vi "rio 9030 2.vi"() -> ()   [LabVIEW 2015]
uses:
  <vilib>/FPGAPlugInAG/cRIO-9030/niLvFpga_Open_cRIO-9030.vi
  <vilib>/rvi/interface/common/dynamic/niFpgaDynamicAddResources.vi
  <vilib>/FPGAPlugInAG/Dynamic/niLvFpga_Abort_Dynamic.vi
  <vilib>/FPGAPlugInAG/Dynamic/niLvFpga_Run_Dynamic.vi
  rio_Global.vi
  <vilib>/Utility/error.llb/Error Cluster From Error Code.vi
  <vilib>/rvi/errors/niLvFpgaAdjustHostInterfaceError.vi
  <vilib>/Analysis/Matrix/Numeric/Conversions/Array To Matrix - RA2.vi
  <vilib>/Analysis/Matrix/Numeric/Multiply/Multiply - RM,RM.vi
  <vilib>/Analysis/Matrix/Numeric/Add/Add - RM,RM.vi
  <vilib>/Analysis/baseanly.llb/Real Inverse Matrix.vi
  <vilib>/Analysis/Matrix/Numeric/Subtract/Subtract - RM,RM.vi
  <vilib>/Analysis/Matrix/Numeric/Conversions/Array To Matrix - RA.vi
  <vilib>/Analysis/Matrix/Numeric/Multiply/Multiply - R,RM.vi
  <vilib>/Analysis/Matrix/Numeric/Conversions/Matrix To Array - RM.vi
  <vilib>/rvi/interface/nirviOpenFPGA/nirviOpenFPGA.xnode
  FPGA Bitfiles/autonomous_FPGATarget4_fpga1_rudp+OsNkSQ.lvbitx
  samsung/fpga 1.vi
  <vilib>/rvi/interface/nirviMethod/nirviMethod.xnode
  <vilib>/rvi/interface/nirviReadWriteControl/nirviReadWriteControl.xnode
  <vilib>/FPGAPlugInAG/Dynamic/niLvFpga_ReadFifo_Dynamic.vi
  <vilib>/rvi/errors/niLvFpgaMergeErrorWithErrorCode.vi
  <vilib>/Analysis/Matrix/NI_Matrix.lvlib
  <vilib>/Analysis/NI_AALBase.lvlib
  <vilib>/rvi/interface/Simulation/niFpgaSimulationCallBeginRW.vi
  NiFpgaLv.dll
  <vilib>/addons/control/pid/NI_PID_pid.lvlib
  <vilib>/ptbypt/NI_PtbyPt.lvlib
  <vilib>/addons/control/pid/pid.llb/PID (DBL).vi
panel:
  in  "steering torque":dbl min=-1.0 max=1.0 step=0.1
  in  "map name":T1(ring)=enum."KAIST"
  out "Waveform Chart 3":dbl(graph)
  in  "lpf gain 2":dbl=0.8 format="%#_13g"
  out "con_dt":dbl
  in  "lpf gain":dbl=0.8 format="%#_13g"
  in  "d gain":dbl=0.003
  out "Waveform Chart 2":dbl(graph)
  in  "Dial":dbl(knob) min=-360.0 max=360.0 step=5.0 scale=-360.0..360.0
  in  "i gain":dbl=6.5
  in  "p gain":dbl=0.02
  out "FPGA":refnum<k20>
  out "C_yaw_rate":dbl
  in  "speed control":bool
  out "C_MCP":dbl
  out "C_APV":dbl
  in  "PWM GAS 2":dbl=1000.0 min=1000.0 max=2000.0 step=1.0
  out "Ref_VS":dbl
  out "XY Graph":cluster{"Y":dbl[], "Y":dbl[]}[](graph)=[{"Y"=[1.82421875, 1.8301353427767753, 1.835194070339203, 1.8394013252854347, 1.8427635002136231, 1.84528698772192, 1.8469781804084777, 1.8478434708714486, 1.8478892517089844, 1.8471219155192375, 1.84554785490036, 1.8431734624505043, 1.8400051307678222, 1.8360492524504661, 1.8313122200965881, 1.8258004263043404, 1.819520263671875, 1.8124781247973443, 1.8046804022789003, 1.796133488714695, 1.7868437767028809, 1.77681765884161, 1.7660615277290344, 1.7545817759633064, 1.742384796142578, 1.7294769808650017, 1.7158647227287291, 1.701554414331913, 1.686552448272705, 1.6708652171492577, 1.654499113559723, 1.637460530102253, 1.619755859375, 1.6013914939761162, 1.5823738265037537, 1.5627092495560646, 1.5424041557312012, 1.5214649376273155, 1.4998979878425598, 1.4777096989750862, 1.4549064636230469, 1.431494674384594, 1.4074807238578795, 1.3828710046410562, 1.3576719093322753, 1.3318898305296898, 1.3055311608314515, 1.2786022928357124, 1.251109619140625, 1.2230595323443412], "Y"=[0.0, 0.5, 1.0, 1.5, 2.0, 2.5, 3.0, 3.5, 4.0, 4.5, 5.0, 5.5, 6.0, 6.5, 7.0, 7.5, 8.0, 8.5, 9.0, 9.5, 10.0, 10.5, 11.0, 11.5, 12.0, 12.5, 13.0, 13.5, 14.0, 14.5, 15.0, 15.5, 16.0, 16.5, 17.0, 17.5, 18.0, 18.5, 19.0, 19.5, 20.0, 20.5, 21.0, 21.5, 22.0, 22.5, 23.0, 23.5, 24.0, 24.5]}, {"Y"=[-1.22265625, -1.2167396572232247, -1.211680929660797, -1.2074736747145653, -1.2041114997863769, -1.20158801227808, -1.1998968195915223, -1.1990315291285514, -1.1989857482910156, -1.1997530844807625, -1.20132714509964, -1.2037015375494957, -1.2068698692321778, -1.2108257475495339, -1.2155627799034119, -1.2210745736956596, -1.227354736328125, -1.2343968752026557, -1.2421945977210997, -1.250741511285305, -1.2600312232971191, -1.27005734115839, -1.2808134722709656, -1.2922932240366936, -1.304490203857422, -1.3173980191349983, -1.3310102772712709, -1.345320585668087, -1.360322551727295, -1.3760097828507423, -1.392375886440277, -1.409414469897747, -1.427119140625, -1.4454835060238838, -1.4645011734962463, -1.4841657504439354, -1.5044708442687988, -1.5254100623726845, -1.5469770121574402, -1.5691653010249138, -1.5919685363769531, -1.615380325615406, -1.6393942761421205, -1.6640039953589438, -1.6892030906677247, -1.7149851694703102, -1.7413438391685485, -1.7682727071642876, -1.795765380859375, -1.8238154676556588, -1.8524165749549866, -1.8815623101592065, -1.911246280670166, -1.9414620938897134, -1.972203357219696, -2.003463678061962, -2.0352366638183597, -2.0675159218907355, -2.1002950596809384, -2.1335676845908162, -2.167327404022217, -2.2015678253769875, -2.2362825560569766, -2.2714652034640315, -2.307109375, -2.3432086780667305, -2.3797567200660703, -2.4167471083998677, -2.4541734504699706, -2.4920293536782263, -2.530308425426483, -2.5690042731165885, -2.6081105041503907, -2.647620725929737, -2.687528545856476, -2.7278275713324547, -2.7685114097595216, -2.809573668539524, -2.8510079550743104, -2.892807876765728, -2.934967041015625, -2.977479055225849, -3.020337526798248, -3.0635360631346704, -3.107068271636963, -3.150927759706974, -3.1951081347465515, -3.2396030041575434, -3.284405975341797, -3.3295106557011604, -3.3749106526374817, -3.4205995735526087, -3.466571025848389, -3.51281861692667, -3.5593359541893004], "Y"=[0.0, 0.5, 1.0, 1.5, 2.0, 2.5, 3.0, 3.5, 4.0, 4.5, 5.0, 5.5, 6.0, 6.5, 7.0, 7.5, 8.0, 8.5, 9.0, 9.5, 10.0, 10.5, 11.0, 11.5, 12.0, 12.5, 13.0, 13.5, 14.0, 14.5, 15.0, 15.5, 16.0, 16.5, 17.0, 17.5, 18.0, 18.5, 19.0, 19.5, 20.0, 20.5, 21.0, 21.5, 22.0, 22.5, 23.0, 23.5, 24.0, 24.5, 25.0, 25.5, 26.0, 26.5, 27.0, 27.5, 28.0, 28.5, 29.0, 29.5, 30.0, 30.5, 31.0, 31.5, 32.0, 32.5, 33.0, 33.5, 34.0, 34.5, 35.0, 35.5, 36.0, 36.5, 37.0, 37.5, 38.0, 38.5, 39.0, 39.5, 40.0, 40.5, 41.0, 41.5, 42.0, 42.5, 43.0, 43.5, 44.0, 44.5, 45.0, 45.5, 46.0, 46.5, 47.0]}, {"Y"=[-0.94, 0.94, 0.94, -0.94, -0.94], "Y"=[-3.2, -3.2, 1.5, 1.5, -3.2]}, {"Y"=[1.984375, 1.978057861328125, 1.9718017578125, 1.965606689453125, 1.95947265625], "Y"=[0.0, 0.5, 1.0, 1.5, 2.0]}, {"Y"=[-5.28125, -5.267578125, -5.25390625, -5.240234375, -5.2265625], "Y"=[0.0, 0.5, 1.0, 1.5, 2.0]}]
  out "x_view":dbl[](array[numeric])=[0.0, 0.5, 1.0, 1.5, 2.0, 2.5, 3.0, 3.5, 4.0, 4.5, 5.0, 5.5, 6.0, 6.5, 7.0, 7.5, 8.0, 8.5, 9.0, 9.5, 10.0, 10.5, 11.0, 11.5, 12.0, 12.5, 13.0, 13.5, 14.0, 14.5, 15.0, 15.5, 16.0, 16.5, 17.0, 17.5, 18.0, 18.5, 19.0, 19.5, 20.0, 20.5, 21.0, 21.5, 22.0, 22.5, 23.0, 23.5, 24.0, 24.5, 25.0, 25.5, 26.0, 26.5, 27.0, 27.5, 28.0, 28.5, 29.0, 29.5, 30.0, 30.5, 31.0, 31.5, 32.0, 32.5, 33.0, 33.5, 34.0, 34.5, 35.0, 35.5, 36.0, 36.5, 37.0, 37.5, 38.0, 38.5, 39.0, 39.5, 40.0, 40.5, 41.0, 41.5, 42.0, 42.5, 43.0, 43.5, 44.0, 44.5, 45.0, 45.5, 46.0, 46.5, 47.0, 47.5, 48.0, 48.5, 49.0, 49.5, 50.0, 50.5, 51.0, 51.5, 52.0, 52.5, 53.0, 53.5, 54.0, 54.5, 55.0, 55.5, 56.0, 56.5, 57.0, 57.5, 58.0, 58.5, 59.0, 59.5, 60.0, 60.5, 61.0, 61.5, 62.0, 62.5, 63.0, 63.5, 64.0, 64.5, 65.0, 65.5, 66.0, 66.5, 67.0, 67.5, 68.0, 68.5, 69.0, 69.5, 70.0, 70.5, 71.0, 71.5, 72.0, 72.5, 73.0, 73.5, 74.0, 74.5, 75.0, 75.5, 76.0, 76.5, 77.0, 77.5, 78.0, 78.5, 79.0, 79.5, 80.0, 80.5, 81.0, 81.5, 82.0, 82.5, 83.0, 83.5, 84.0, 84.5, 85.0, 85.5, 86.0, 86.5, 87.0, 87.5, 88.0, 88.5, 89.0, 89.5, 90.0, 90.5, 91.0, 91.5, 92.0, 92.5, 93.0, 93.5, 94.0, 94.5, 95.0, 95.5, 96.0, 96.5, 97.0, 97.5, 98.0, 98.5, 99.0, 99.5, 100.0, 100.5, 101.0, 101.5, 102.0, 102.5, 103.0, 103.5, 104.0, 104.5, 105.0, 105.5, 106.0, 106.5, 107.0, 107.5, 108.0, 108.5, 109.0, 109.5, 110.0, 110.5, 111.0, 111.5, 112.0, 112.5, 113.0, 113.5, 114.0, 114.5, 115.0, 115.5, 116.0, 116.5, 117.0, 117.5, 118.0, 118.5, 119.0, 119.5, 120.0, 120.5, 121.0, 121.5, 122.0, 122.5, 123.0, 123.5, 124.0, 124.5, 125.0, 125.5, 126.0, 126.5, 127.0, 127.5, 128.0]
  in  "Manual Steering torque":dbl(slide) min=-0.9 max=0.9 step=0.01 scale=-0.9..0.9
  out "T init":i32
  out "T out":i32
  out "PWM GAS":dbl=1000.0 min=1000.0 max=2000.0 step=1.0
  out "Mobileye_time 50":u32
  out "H_GPS":dbl
  out "vgain":dbl=1.0
  out "vcount":u64=1
  out "hbias":dbl
  out "hcount":u64=1
  out "get heading":bool
  out "get position":bool
  out "heading error":dbl
  out "h_gps":dbl
  out "rt":dbl
  out "pos error":dbl
  out "POS init":bool
  out "Heading":dbl
  out "pos":dbl[](array[numeric])
  in  "GPS init":bool=TRUE
  out "pos_gps":dbl[](array[numeric]) format="%#_19f"
  out "dt":dbl
  out "Pos_time 10":i32
  out "map":i32=2
  out "ecef ref":dbl[](array[numeric])
  in  "Velocity input":bool
  in  "Manual Speed":dbl=20.0
  in  "Steer input":bool=TRUE
  out "Run":bool
  out "Auto":bool
  out "E - STOP":bool
  out "Con_time 10":i32
  out "VS_CAN":dbl
  out "CAN_time 10":u32
  out "gps1":refnum<visa-resource-name>
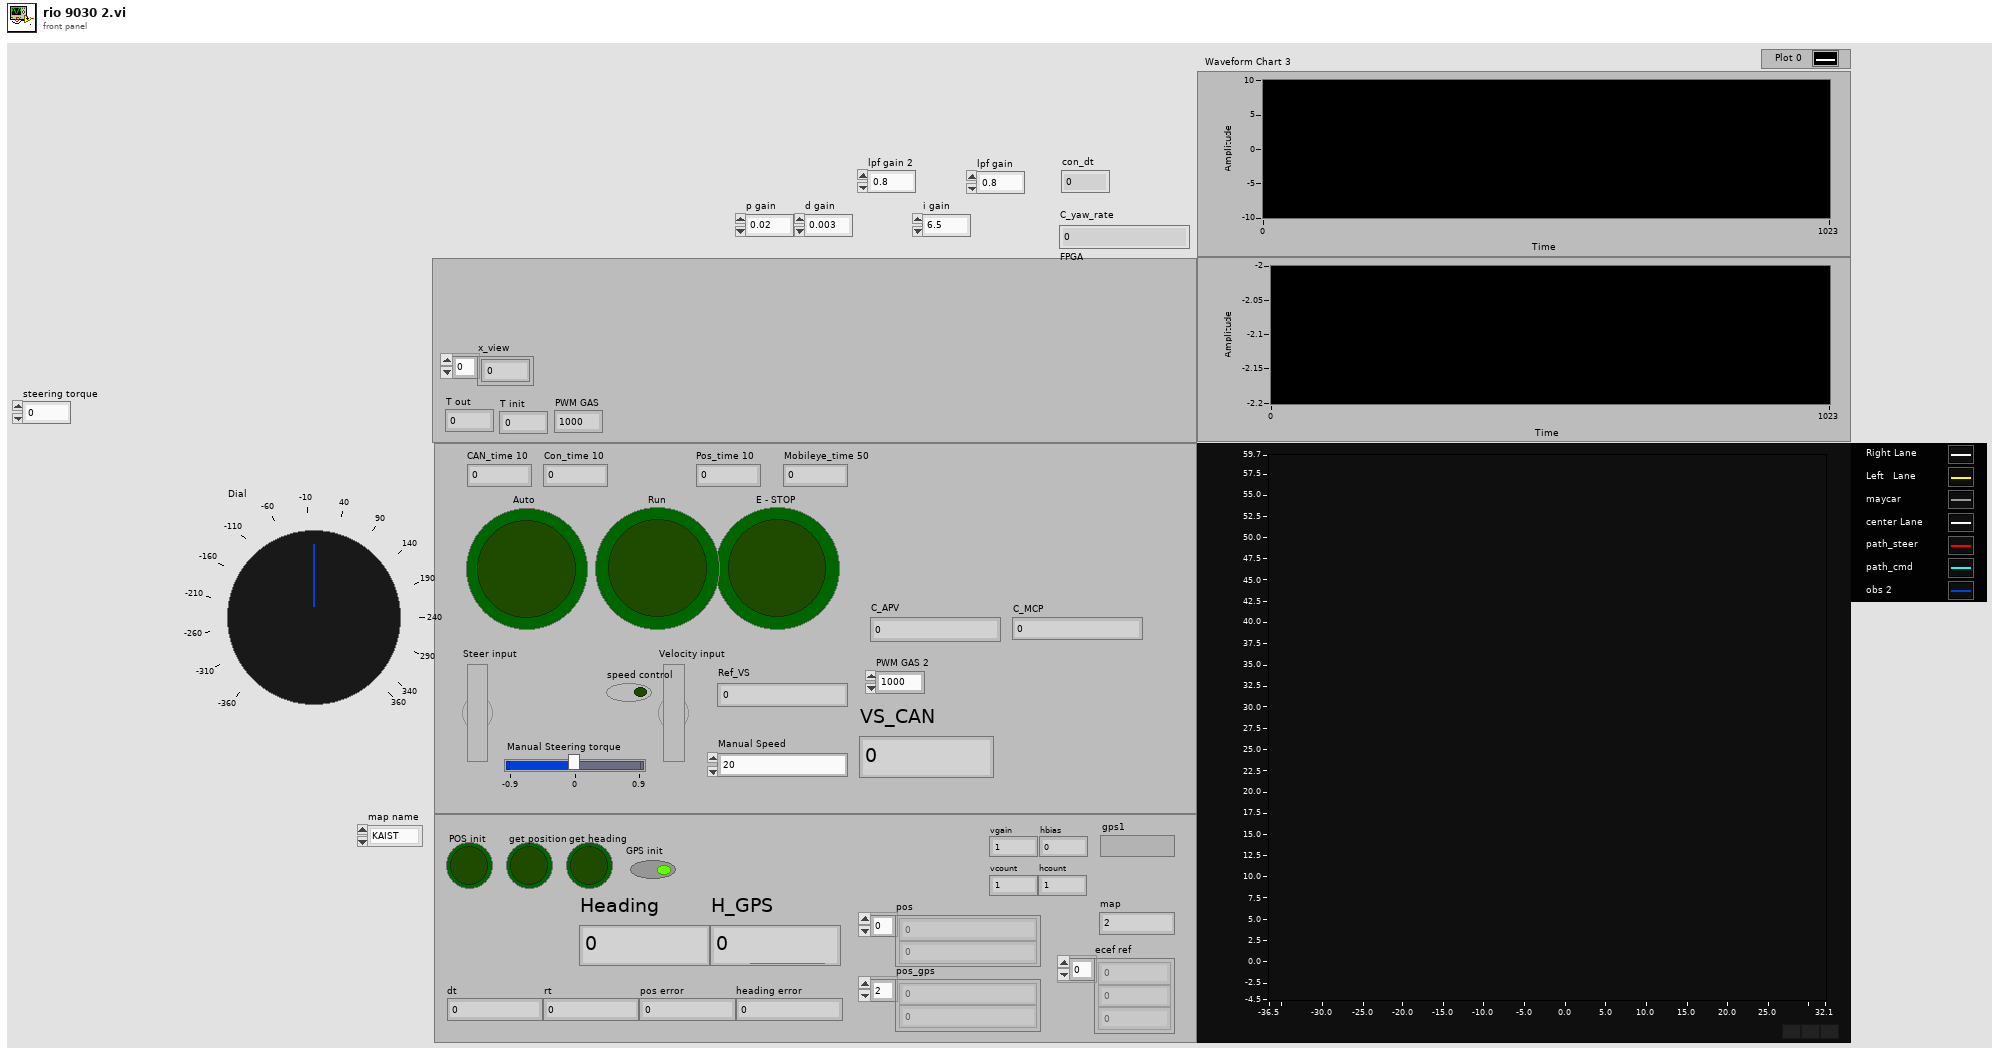
[diagram p1: front panel]
types:
  T1 = enum32{"Namyang", "Hyundai", "KAIST", "Ajou", "Munji", "Airforce", "Car", "KATRI", "Samsung", "Coex", "Gwangnaru", "Inje", "sinjin"}
  T2 = cluster{"identifier":u32, "timestamp":timestamp, "payload":u8[]}
  T3 = cluster{"timestamp high":u32, "timestamp low":u32, "identifier":u32, "type":enum8{"Data Frame", "Remote Frame", "(reserved)", "(reserved) ", "(reserved)  ", "(reserved)   ", "Bus Error", "Transceiver Fault"}, "info A":u8, "info B":u8, "data length":u8, "data":u8[]}
  T4 = cluster{"connection ID":refnum<k16>, "net address":u32, "port":u16}
  T5 = cluster{"hash":i64, "sys time":i64, "size":i32, "data":u8[]}
  T6 = cluster{"hash":i64, "sys time":i64, "time":dbl, "yaw_rate":dbl, "mdps torque":dbl, "mdps str_ang":dbl, "VS_CAN":dbl, "lat_accel":dbl, "mcp":dbl, "accel pedal value":dbl, "tps":dbl, "odometer":dbl, "battery voltage":dbl, "WHL_SPD_RR":dbl, "WHL_SPD_RL":dbl, "WHL_SPD_FR":dbl, "WHL_SPD_FL":dbl}
  T7 = cluster{"proportional gain (Kc)":dbl, "integral time (Ti, min)":dbl, "derivative time (Td, min)":dbl}
  T8 = cluster{"hash":i64, "sys time":i64, "ref_vel":dbl, "ref_steer":dbl, "alert":u8}
  T9 = cluster{"hash":i64, "sys time":i64, "ref_vel":dbl, "ref_steer":dbl}
  T10 = cluster{"hash":i64, "sys time":i64, "Auto":bool, "Run":bool, "Solenoid":bool, "T lim":bool, "brk_enc":u8, "B PWM":u16, "T PWM":u16, "ref_vel":dbl, "ref_bkr_enc":dbl, "ref_apv":dbl, "ref_steer":dbl, "net address":u32}
  T11 = typedef "NI_Matrix.lvlib/RealMatrix.ctl" = dbl[][]
  T12 = cluster{"hash":i64, "sys time":i64, "dt":dbl, "x":dbl, "y":dbl, "speed":dbl, "heading":dbl, "yaw_rate":dbl}
  T13 = cluster{"Real 2D Array[0]":dbl, "Real 2D Array[1]":dbl, "Real 2D Array[2]":dbl, "Real 2D Array[3]":dbl, "Real 2D Array[4]":dbl}
  T14 = cluster{"hash":i64, "sys time":i64, "time":dbl, "x":dbl, "y":dbl, "h":dbl, "numSV":i32, "postype":i32, "lag":i32, "hordev":dbl, "lat":dbl, "lon":dbl, "hgt":dbl, "map_idx":i32}
  T15 = cluster{"output[0]":dbl, "output[1]":dbl, "output[2]":dbl, "output[3]":dbl, "output[4]":dbl, "output[5]":dbl, "output[6]":dbl, "output[7]":dbl, "output[8]":dbl, "output[9]":dbl, "output[10]":dbl, "output[11]":dbl, "output[12]":dbl, "output[13]":dbl, "output[14]":dbl}
  T16 = cluster{"hash":i64, "sys time":i64, "time":dbl, "speed":dbl, "heading":dbl, "lat":dbl, "lon":dbl}
  T17 = cluster{"output[0]":dbl, "output[1]":dbl, "output[2]":dbl, "output[3]":dbl, "output[4]":dbl, "output[5]":dbl, "output[6]":dbl}
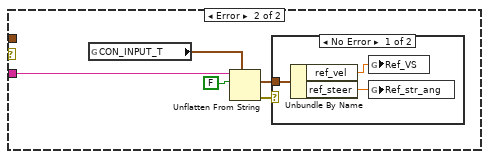
[diagram p3: hidden frame]
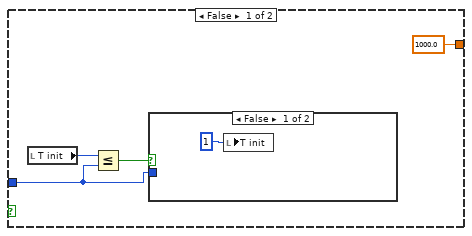
[diagram p5: hidden frame]
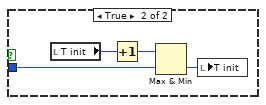
[diagram p6: hidden frame]
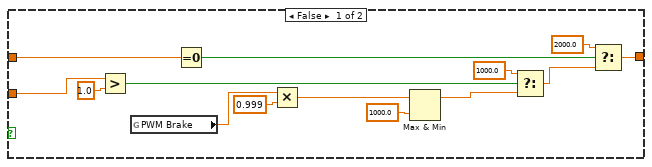
[diagram p8: hidden frame]
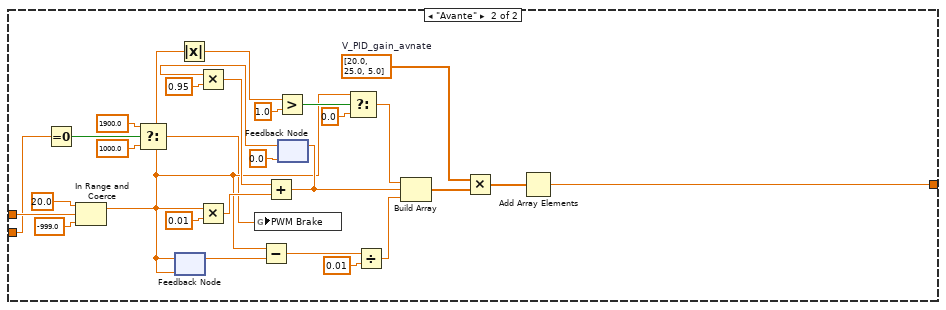
[diagram p9: hidden frame]
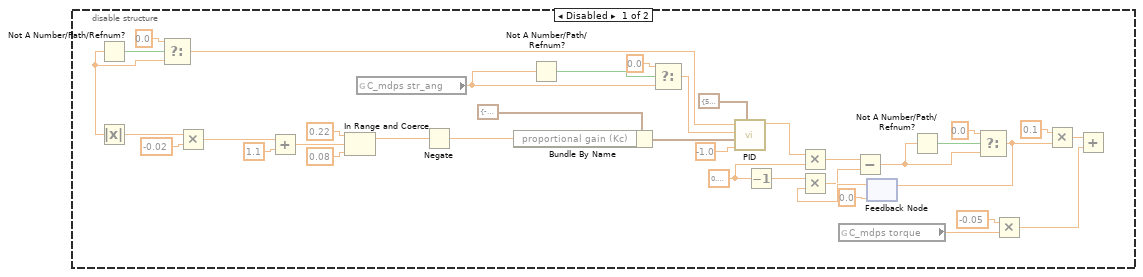
[diagram p10: hidden frame]
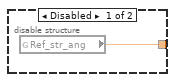
[diagram p14: hidden frame]
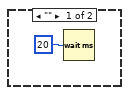
[diagram p15: hidden frame]
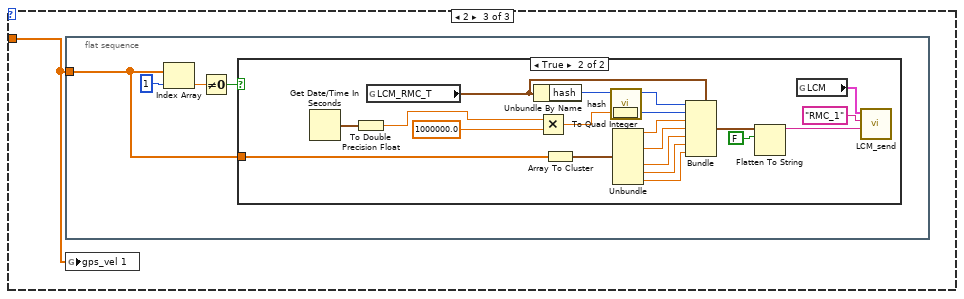
[diagram p18: hidden frame]
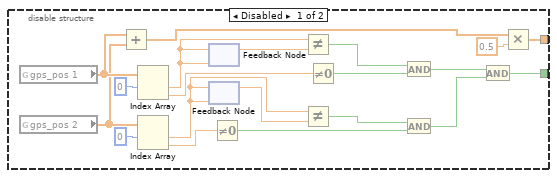
[diagram p20: hidden frame]
diagram:
  n1 = flat-sequence {
    frame #0 {
      n2 = for {
        N: 257 -> [_]
        tunnel: [w8] -> w6 mode=indexing
        i -> [w8]
      }
      n3 = Multiply(x=w6, y=0.5) -> (x*y=w4:dbl[])
      "x_view" <- w4
      n4 = Array Subset(array=w4, index=30) -> (w2:dbl[])  [unwired: 1 in]
      n5 = global write "rio_Global.vi" "x_view"(w2) -> ()
    }
    frame #1 {
      n6 = while {
        stop <- FALSE stop-if-true
        n7 = flat-sequence {
          frame #0 {
            n8 = Wait Until Next ms Multiple(millisecond multiple=u32 33) -> ()  [unwired: 1 out]
          }
          frame #1 {
            n9 = local read "x_view"() -> (w11:dbl[])
            n10 = call "mobileye_disp.vi"("x_view"=w11) -> ("XY Graph"=→"XY Graph":cluster{"Y":dbl[], "Y":dbl[]}[])  [unwired: 10 in]
          }
        }
      }
    }
  }
  n11 = flat-sequence {
    frame #0 {
      w14 = u16 7668 ("port")
      w23 = u16 7667 ("port")
      n12 = disable-structure shown="Enabled" {
        frame Disabled {
        }
        frame Enabled {
          w30 = 0.0 ("Ref_str_ang")
          w31 = 1000.0 ("PWM GAS")
          n13 = global write "rio_Global.vi" "steering torque"(0.0 ("steering")) -> ()
          n14 = global write "rio_Global.vi" "Auto SW"(FALSE ("Auto SW")) -> ()
          n15 = global write "rio_Global.vi" "Solenoid"(FALSE ("CAN A 1")) -> ()
          n16 = global write "rio_Global.vi" "PWM GAS"(w31) -> ()
          n17 = global write "rio_Global.vi" "PWM Brake"(w31) -> ()
          n18 = global write "rio_Global.vi" "Ref_VS"(w30) -> ()
          n19 = global write "rio_Global.vi" "Ref_str_ang"(w30) -> ()
        }
      }
      n20 = xnode "Open FPGA VI Reference"() -> ("FPGA VI Reference Out"=w25:refnum<k20>, "error out"=w26:errorcluster)  [unwired: 2 in]
      n21 = global read "rio_Global.vi" "LCM PC"() -> (w18:T4)
      n22 = Decrement(x=w23) -> (x-1=w24:u16)
      n23 = UDP Open(11:w14) -> (port=w16:refnum<k16>)  [unwired: 4 in, 2 out]
      n24 = xnode "Invoke Method"("FPGA VI Reference In"=w25, "error in"=w26) -> ("FPGA VI Reference Out"=w27:refnum<k20>, "error out"=w28:errorcluster)
      n25 = Bundle By Name(cluster=w18, "port"=w14, "connection ID"=w16, "net address"=u32 0) -> (w17:T4)
      n26 = UDP Open(11:w24) -> (port=w21:refnum<k16>)  [unwired: 4 in, 2 out]
      n27 = xnode "Invoke Method"("FPGA VI Reference In"=w27, "error in"=w28, "Wait Until Done (F)"=FALSE) -> ("FPGA VI Reference Out"=→"FPGA":refnum<k20>)  [unwired: 1 out]
      n28 = global read "rio_Global.vi" "LCM"() -> (w19:T4)
      n29 = global write "rio_Global.vi" "LCM PC"(w17) -> ()
      n30 = Bundle By Name(cluster=w19, "port"=w23, "connection ID"=w21, "net address"=u32 4294967295) -> (w20:T4)
      n31 = global write "rio_Global.vi" "LCM"(w20) -> ()
    }
    frame #1 {
      n32 = while {
        stop <- FALSE stop-if-true
        n33 = flat-sequence {
          tunnel: [w228] -> w222
          tunnel: w222 -> [w251]
          frame #0 {
            n34 = Wait Until Next ms Multiple(millisecond multiple=u32 10) -> ()  [unwired: 1 out]
          }
          frame #1 {
            n35 = global read "rio_Global.vi" "Car_name"() -> (w225:string)
            n36 = local read "FPGA"() -> (w230:refnum<k20>)
            n37 = case shown="Default" w225 {
              tunnel: w230 -> [w233 w240]
              tunnel: [_ w238] -> w229
              tunnel: [w233 w236] -> w228
              tunnel: [w232 w235] -> w227
              tunnel: [w231 w234] -> w226
              frame "Santafe" {
                n38 = global read "rio_Global.vi" "Auto"() -> (w232:bool)
                n39 = global read "rio_Global.vi" "Run"() -> (w231:bool)
              }
              frame Default {
                n40 = xnode "Read/Write Control"("FPGA VI Reference In"=w240) -> ("FPGA VI Reference Out"=w236:refnum<k20>, "Auto"=w235:bool, "Run"=w239:bool)  [unwired: 1 in, 1 out]
                n41 = global write "rio_Global.vi" "Auto"(w235) -> ()
                n42 = And(x=w235, y=w239) -> (x .and. y?=w234:bool)
                n43 = global write "rio_Global.vi" "Run"(w234) -> ()
                n44 = Not(x=w234) -> (.not. x?=w237:bool)
                n45 = And(x=w235, y=w237) -> (x .and. y?=w238:bool)
              }
            }
            "E - STOP" <- w229
            "Auto" <- w227
            "Run" <- w226
          }
          frame #2 {
            w242 = fxp<+/-,20,5> 0.0 ("Mod3/AO3")
            n46 = case shown="True" "speed control" {
              tunnel: [w261 w277] -> w250
              tunnel: [w261 w274] -> w249
              tunnel: [_ w267] -> w248
              frame False {
                w261 = u16 1000
              }
              frame True {
                n47 = disable-structure shown="Enabled" {
                  disable-tunnel: [w283 "PWM GAS 2"] -> w266
                  frame Enabled {
                    n48 = global read "rio_Global.vi" "PWM Brake"() -> (w283:dbl)
                  }
                  frame Disabled {
                  }
                }
                n49 = disable-structure shown="Enabled" {
                  disable-tunnel: [w282 _] -> w279
                  frame Enabled {
                    n50 = global read "rio_Global.vi" "PWM GAS"() -> (w282:dbl)
                  }
                  frame Disabled {
                  }
                }
                n51 = Round To Nearest(number=w266) -> (nearest integer value=w265:dbl)
                n52 = disable-structure shown="Enabled" {
                  disable-tunnel: [w280 TRUE ("Solenoid")] -> w270
                  frame Enabled {
                    n53 = global read "rio_Global.vi" "Solenoid"() -> (w280:bool)
                  }
                  frame Disabled {
                  }
                }
                n54 = Select(t=w265, s=TRUE, f=1900.0 ("t")) -> (s? t:f=w273:dbl)
                n55 = Round To Nearest(number=w279) -> (nearest integer value=w271:dbl)
                n56 = local read "Run"() -> (w263:bool)
                n57 = global read "rio_Global.vi" "Auto"() -> (w276:bool)
                n58 = local read "Run"() -> (w262:bool)
                n59 = Select(t=w271, s=w263, f=1000.0) -> (s? t:f=w268:dbl)
                n60 = Select(t=w273, s=w276, f=1000.0) -> (s? t:f=w269:dbl)
                n61 = To Unsigned Word Integer(number=w268) -> (unsigned 16bit integer=w277:u16)
                n62 = To Unsigned Word Integer(number=w269) -> (unsigned 16bit integer=w274:u16)
                n63 = Select(t=w270, s=w262, f=w262) -> (s? t:f=w267:bool)
              }
            }
            n64 = global read "rio_Global.vi" "Auto"() -> (w241:bool)
            n65 = case shown="True" w241 {
              tunnel: [_ w253] -> w246
              tunnel: [_ w252] -> w245
              frame False {
              }
              frame True {
                n66 = disable-structure shown="Enabled" {
                  disable-tunnel: [w256 "steering torque"] -> w254
                  frame Disabled {
                    n67 = global read "rio_Global.vi" "steering torque"() -> (w256:dbl)
                  }
                  frame Enabled {
                  }
                }
                n68 = Greater Than 0?(x=w254) -> (x > 0?=w255:bool)
                n69 = case shown="True" w255 {
                  tunnel: w254 -> [w259 w260]
                  tunnel: [w258 _] -> w253
                  tunnel: [_ w260] -> w252
                  frame False {
                    n70 = Absolute Value(x=w259) -> (abs(x)=w258:dbl)
                  }
                  frame True {
                  }
                }
              }
            }
            n71 = To Fixed-Point(fixed-point type=w242, number=w246) -> (fixed-point=w244:fxp<+/-,20,5>)
            n72 = To Fixed-Point(fixed-point type=w242, number=w245) -> (fixed-point=w243:fxp<+/-,20,5>)
            n73 = xnode "Read/Write Control"("FPGA VI Reference In"=w251, "Solenoid"=w248, "PWM Gas"=w250, "PWM Brake"=w249, "Mod3/AO0"=w244, "Mod3/AO1"=w243) -> ()  [unwired: 1 in, 2 out]
          }
        }
      }
      n74 = flat-sequence {
        tunnel: [w109] -> w40
        tunnel: w40 -> [w117]
        tunnel: [w117] -> w39
        tunnel: w39 -> [w119]
        tunnel: [w122] -> w38
        tunnel: [w142] -> w37
        tunnel: w38 -> [w142]
        tunnel: [w143] -> w36
        tunnel: w37 -> [w144]
        tunnel: w36 -> [w146]
        frame #0 {
          n75 = local read "FPGA"() -> (w115:refnum<k20>)
          n76 = xnode "Invoke Method"("FPGA VI Reference In"=w115, "Number of Elements"=u32 0, "Timeout (ms)"=0) -> ("FPGA VI Reference Out"=w113:refnum<k20>, "Elements Remaining"=w114:u32)  [unwired: 1 in, 2 out]
          n77 = xnode "Invoke Method"("FPGA VI Reference In"=w113, "Number of Elements"=w114, "Timeout (ms)"=0) -> ("FPGA VI Reference Out"=w109:refnum<k20>)  [unwired: 1 in, 3 out]
        }
        frame #1 {
          n78 = Wait (ms)(milliseconds to wait=u32 100) -> ()  [unwired: 1 out]
        }
        frame #2 {
          n79 = xnode "Read/Write Control"("FPGA VI Reference In"=w119, "send can 1"=TRUE) -> ("FPGA VI Reference Out"=w118:refnum<k20>)  [unwired: 1 in, 1 out]
          n80 = for {
            N: 100 -> [_]
            tunnel: w118 -> [w125]
            tunnel: [w127] -> w122
            i -> [w124]
            n81 = Split Number(x=u16 65535 ("y")) -> (hi(x)=w136:u8, lo(x)=w135:u8)
            n82 = To Unsigned Byte Integer(number=w124) -> (unsigned 8bit integer=w123:u8)
            n83 = Build Array(u8 0 ("Con steer status"), w135, w136, u8 0 ("element"), w123, u8 0 ("element"), u8 0 ("element")) -> (w130:u8[])
            n84 = Add Array Elements(numeric array=w130) -> (sum=w131:u8)
            n85 = Build Array (concatenate)(w130, w131) -> (w128:u8[])
            n86 = Bundle By Name(cluster=T3 {"timestamp high"=0, "timestamp low"=0, "identifier"=0, "type"=enum."Data Frame", "info A"=0, "info B"=0, "data length"=8, "data"=[0, 0, 0, 0, 0, 0, 0, 0]} ("Mod4/CAN1 input"), "identifier"=u32 912, "data"=w128, "data length"=u8 8) -> (w137:T3)
            n87 = xnode "Read/Write Control"("FPGA VI Reference In"=w125, "Mod2/CAN1 input"=w137) -> ("FPGA VI Reference Out"=w127:refnum<k20>)  [unwired: 1 in, 1 out]
          }
        }
        frame #3 {
          n88 = Wait (ms)(milliseconds to wait=u32 100) -> ()  [unwired: 1 out]
        }
        frame #4 {
          n89 = xnode "Read/Write Control"("FPGA VI Reference In"=w144, "send can 1"=FALSE) -> ("FPGA VI Reference Out"=w143:refnum<k20>)  [unwired: 1 in, 1 out]
        }
        frame #5 {
          n90 = while {
            tunnel: w146 -> [w147]
            stop <- FALSE stop-if-true
            n91 = flat-sequence {
              tunnel: [w150] -> w148
              tunnel: w147 -> [w150]
              tunnel: w148 -> [w157]
              frame #0 {
                n92 = Wait Until Next ms Multiple(millisecond multiple=u32 10) -> (millisecond timer value=w153:u32)
                n93 = feedback #1(w153) -> (w152:u32)
                n94 = feedback-in #1(w153) -> ()
                n95 = Subtract(x=w153, y=w152) -> (x-y=→"CAN_time 10":u32)
              }
              frame #1 {
                n96 = while {
                  tunnel: w157 -> [w218]
                  tunnel: [w215] -> w156 mode=indexing
                  stop <- w214 stop-if-true
                  n97 = xnode "Invoke Method"("FPGA VI Reference In"=w218, "Number of Elements"=u32 16, "Timeout (ms)"=0) -> ("FPGA VI Reference Out"=w213:refnum<k20>, "Data"=w215:u8[], "Elements Remaining"=w210:u32)  [unwired: 1 in, 1 out]
                  n98 = Equal To 0?(x=w210) -> (x = 0?=w214:bool)
                  n99 = Quotient & Remainder(x=w210, y=u32 16) -> (x-y*floor(x/y)=w211:u32)  [unwired: 1 out]
                  n100 = case shown="1, Default" w211 {
                    selector: w211 -> [w221 _]
                    tunnel: w213 -> [w220 _]
                    frame 1, Default {
                      n101 = xnode "Invoke Method"("FPGA VI Reference In"=w220, "Number of Elements"=w221, "Timeout (ms)"=0) -> ()  [unwired: 1 in, 4 out]
                    }
                    frame 0 {
                    }
                  }
                }
                n102 = Empty Array?(array=w156) -> (empty?=w155:bool)
                n103 = case shown="False" w155 {
                  tunnel: w156 -> [w160 _]
                  frame False {
                    n104 = flat-sequence {
                      tunnel: w160 -> [w161]
                      tunnel: [w161] -> w159
                      tunnel: w159 -> [w194]
                      tunnel: [w179] -> w158
                      tunnel: w158 -> [w202]
                      frame #0 {
                        n105 = for {
                          tunnel: w161 -> [w171] mode=indexing
                          w174 = 4 ("length")
                          w172 = 8 ("index")
                          n106 = Delete From Array(array=w171, length=w172, index=w172) -> (deleted portion=w163:u8[], array with subset deleted=w173:u8[])
                          n107 = Delete From Array(array=w173, length=w174, index=w174) -> (deleted portion=w178:u8[], array with subset deleted=w175:u8[])
                          n108 = Type Cast(type=u32 0, x=w175) -> (*(type *) &x=w164:u32)
                          n109 = Type Cast(type=u32 0, x=w178) -> (*(type *) &x=w165:u32)
                          n110 = Multiply(x=w165, y=1e-07) -> (x*y=w168:dbl)
                          n111 = To Time Stamp(1:w168) -> (0:w167:timestamp)
                          n112 = Bundle By Name(cluster=T2 {"identifier"=0, "timestamp"=timestamp(0 s since 1904-01-01), "payload"=[]} ("can cluster"), "identifier"=w164, "payload"=w163, "timestamp"=w167) -> (w170:T2)
                          n113 = global read "rio_Global.vi" "Car_name"() -> (w162:string)
                          n114 = call "can decoder.vi"("can cluster"=w170, "name"=w162) -> ()  [unwired: 10 in]
                        }
                      }
                      frame #1 {
                        n115 = Array Size(array=w194) -> (size(s)=w195:i32[])
                        n116 = global read "rio_Global.vi" "LCM_CAN_RAW_SNAP"() -> (w192:T5)
                        n117 = Multiply Array Elements(1:w195) -> (0:w186:i32)
                        n118 = Get Date/Time In Seconds() -> (seconds since 1Jan1904=w190:timestamp)
                        n119 = To Double Precision Float(number=w190) -> (double precision float=w189:dbl)
                        n120 = Reshape Array(w194, w186) -> (w185:u8[])
                        n121 = Unbundle By Name(w192) -> ("hash"=w187:i64)
                        n122 = Multiply(x=w189, y=1000000.0) -> (x*y=w191:dbl)
                        n123 = call "hash.vi"("input"=w187) -> ("output"=w193:i64)  [unwired: 10 in]
                        n124 = To Quad Integer(1:w191) -> (0:w179:i64)
                        n125 = Bundle(cluster=w192, "hash"=w193, "sys time"=w179, "size"=w186, "data"=w185) -> (w183:T5)
                        n126 = global read "rio_Global.vi" "Car_name"() -> (w180:string)
                        n127 = Flatten To String(anything=w183, prepend array or string size? (T)=FALSE) -> (data string=w181:string)  [unwired: 2 in, 2 out]
                        n128 = global read "rio_Global.vi" "LCM"() -> (w182:T4)
                        n129 = call "LCM_send.vi"("DATA"=w181, "ID"=w180, "LCM"=w182) -> ()  [unwired: 7 in, 2 out]
                      }
                      frame #2 {
                        n130 = global read "rio_Global.vi" "LCM_CAN_T"() -> (w208:T6)
                        n131 = global read "rio_Global.vi" "C_time"() -> (w204:u32)
                        n132 = global read "rio_Global.vi" "C_mdps str_ang"() -> (w206:dbl)
                        n133 = global read "rio_Global.vi" "C_mdps torque"() -> (w196:dbl)
                        n134 = Unbundle By Name(w208) -> ("hash"=w209:i64)
                        n135 = global read "rio_Global.vi" "C_VS_CAN"() -> (w205:dbl)
                        n136 = call "hash.vi"("input"=w209) -> ("output"=w207:i64)  [unwired: 10 in]
                        n137 = To Double Precision Float(number=w204) -> (double precision float=w203:dbl)
                        n138 = Bundle By Name(cluster=w208, "hash"=w207, "mdps str_ang"=w206, "time"=w203, "VS_CAN"=w205, "sys time"=w202, "mdps torque"=w196) -> (w199:T6)
                        n139 = Flatten To String(anything=w199, prepend array or string size? (T)=FALSE) -> (data string=w198:string)  [unwired: 2 in, 2 out]
                        n140 = global read "rio_Global.vi" "LCM"() -> (w201:T4)
                        n141 = call "LCM_send.vi"("DATA"=w198, "ID"="CAN_T", "LCM"=w201) -> ()  [unwired: 7 in, 2 out]
                      }
                    }
                  }
                  frame True {
                  }
                }
              }
            }
          }
        }
      }
      n142 = flat-sequence {
        tunnel: [w41] -> w35
        tunnel: w35 -> [w48]
        frame #0 {
          n143 = local read "FPGA"() -> (w42:refnum<k20>)
          n144 = xnode "Invoke Method"("FPGA VI Reference In"=w42, "Number of Elements"=u32 0, "Timeout (ms)"=0) -> ("FPGA VI Reference Out"=w44:refnum<k20>, "Elements Remaining"=w45:u32)  [unwired: 1 in, 2 out]
          n145 = xnode "Invoke Method"("FPGA VI Reference In"=w44, "Number of Elements"=w45, "Timeout (ms)"=0) -> ("FPGA VI Reference Out"=w41:refnum<k20>)  [unwired: 1 in, 3 out]
        }
        frame #1 {
          n146 = while {
            tunnel: w48 -> [w49]
            stop <- FALSE stop-if-true
            n147 = flat-sequence {
              tunnel: [w52] -> w50
              tunnel: w49 -> [w52]
              tunnel: w50 -> [w59]
              frame #0 {
                n148 = Wait Until Next ms Multiple(millisecond multiple=u32 50) -> (millisecond timer value=w54:u32)
                n149 = feedback #2(w54) -> (w55:u32)
                n150 = feedback-in #2(w54) -> ()
                n151 = Subtract(x=w54, y=w55) -> (x-y=→"Mobileye_time 50":u32)
              }
              frame #1 {
                n152 = while {
                  tunnel: w59 -> [w105]
                  tunnel: [w102] -> w58 mode=indexing
                  stop <- w100 stop-if-true
                  n153 = xnode "Invoke Method"("FPGA VI Reference In"=w105, "Number of Elements"=u32 16, "Timeout (ms)"=0) -> ("FPGA VI Reference Out"=w101:refnum<k20>, "Data"=w102:u8[], "Elements Remaining"=w99:u32)  [unwired: 1 in, 1 out]
                  n154 = Equal To 0?(x=w99) -> (x = 0?=w100:bool)
                  n155 = Quotient & Remainder(x=w99, y=u32 16) -> (x-y*floor(x/y)=w97:u32)  [unwired: 1 out]
                  n156 = case shown="1, Default" w97 {
                    selector: w97 -> [w108 _]
                    tunnel: w101 -> [w107 _]
                    frame 1, Default {
                      n157 = xnode "Invoke Method"("FPGA VI Reference In"=w107, "Number of Elements"=w108, "Timeout (ms)"=0) -> ()  [unwired: 1 in, 4 out]
                    }
                    frame 0 {
                    }
                  }
                }
                n158 = Empty Array?(array=w58) -> (empty?=w57:bool)
                n159 = case shown="False" w57 {
                  tunnel: w58 -> [w61 _]
                  frame False {
                    n160 = flat-sequence {
                      tunnel: w61 -> [w62]
                      tunnel: [w62] -> w60
                      tunnel: w60 -> [w81]
                      frame #0 {
                        n161 = for {
                          tunnel: w62 -> [w72] mode=indexing
                          w75 = 4 ("length")
                          w73 = 8 ("index")
                          n162 = Delete From Array(array=w72, length=w73, index=w73) -> (deleted portion=w63:u8[], array with subset deleted=w74:u8[])
                          n163 = Delete From Array(array=w74, length=w75, index=w75) -> (deleted portion=w79:u8[], array with subset deleted=w76:u8[])
                          n164 = Type Cast(type=u32 0, x=w76) -> (*(type *) &x=w64:u32)
                          n165 = Type Cast(type=u32 0, x=w79) -> (*(type *) &x=w65:u32)
                          n166 = Multiply(x=w65, y=1e-07) -> (x*y=w70:dbl)
                          n167 = To Time Stamp(1:w70) -> (0:w68:timestamp)
                          n168 = Bundle By Name(cluster=T2 {"identifier"=0, "timestamp"=timestamp(0 s since 1904-01-01), "payload"=[]} ("can cluster"), "identifier"=w64, "payload"=w63, "timestamp"=w68) -> (w66:T2)
                          n169 = call "mobileye_decoder.vi"("can cluster"=w66, "name"="Mobileye560") -> ()  [unwired: 10 in]
                        }
                      }
                      frame #1 {
                        n170 = Array Size(array=w81) -> (size(s)=w82:i32[])
                        n171 = global read "rio_Global.vi" "LCM_CAN_RAW_SNAP"() -> (w85:T5)
                        n172 = Multiply Array Elements(1:w82) -> (0:w91:i32)
                        n173 = Get Date/Time In Seconds() -> (seconds since 1Jan1904=w87:timestamp)
                        n174 = To Double Precision Float(number=w87) -> (double precision float=w88:dbl)
                        n175 = Reshape Array(w81, w91) -> (w92:u8[])
                        n176 = Unbundle By Name(w85) -> ("hash"=w90:i64)
                        n177 = Multiply(x=w88, y=1000000.0) -> (x*y=w86:dbl)
                        n178 = To Quad Integer(1:w86) -> (0:w83:i64)
                        n179 = call "hash.vi"("input"=w90) -> ("output"=w84:i64)  [unwired: 10 in]
                        n180 = Bundle(cluster=w85, "hash"=w84, "sys time"=w83, "size"=w91, "data"=w92) -> (w94:T5)
                        n181 = Flatten To String(anything=w94, prepend array or string size? (T)=FALSE) -> (data string=w96:string)  [unwired: 2 in, 2 out]
                        n182 = global read "rio_Global.vi" "LCM"() -> (w95:T4)
                        n183 = call "LCM_send.vi"("DATA"=w96, "ID"="Mobileye560" ("name"), "LCM"=w95) -> ()  [unwired: 7 in, 2 out]
                      }
                    }
                  }
                  frame True {
                  }
                }
              }
            }
          }
        }
      }
    }
  }
  n184 = flat-sequence {
    frame #0 {
      w289 = "Avante" ("Car_name")
      n185 = local write "Manual Steering torque"(0.0 ("Ref_vel_planner")) -> ()
      n186 = local write "Steer input"(FALSE ("Steer input")) -> ()
      n187 = global write "rio_Global.vi" "Car_name"(w289) -> ()
      n188 = local write "Manual Speed"(20.0 ("manual Speed")) -> ()
      n189 = local write "Velocity input"(FALSE ("GPS init")) -> ()
      n190 = call "car_spec.vi"("Car_name"=w289) -> ("turn radius"=w285:dbl, "wheel base"=w286:dbl, "ratio"=w287:dbl, "overall width"=w288:dbl)  [unwired: 5 in, 2 out]
      n191 = global write "rio_Global.vi" "overall width"(w288) -> ()
      n192 = global write "rio_Global.vi" "ratio"(w287) -> ()
      n193 = global write "rio_Global.vi" "wheel base"(w286) -> ()
      n194 = global write "rio_Global.vi" "turn radius"(w285) -> ()
    }
    frame #1 {
      n195 = while {
        stop <- FALSE stop-if-true
        n196 = flat-sequence {
          frame #0 {
            n197 = Wait Until Next ms Multiple(millisecond multiple=u32 10) -> (millisecond timer value=w298:u32)
            n198 = feedback #3(w298) -> (w297:u32)
            n199 = feedback-in #3(w298) -> ()
            n200 = Subtract(x=w298, y=w297) -> (x-y=w296:u32)
            n201 = To Long Integer(number=w296) -> (32bit integer=→"Con_time 10":i32)
          }
          frame #1 {
            n202 = global read "rio_Global.vi" "LCM PC"() -> (w302:T4)
            n203 = call "LCM_read.vi"("LCM"=w302) -> ("data"=w300:string, "ID"=w301:string)  [unwired: 7 in, 2 out]
            n204 = case shown="\"CON_INPUT_T\"" w301 {
              tunnel: w300 -> [_ w303]
              frame "False", Default {
              }
              frame "CON_INPUT_T" {
                n205 = global read "rio_Global.vi" "CON_INPUT_T 2"() -> (w305:T8)
                n206 = Unflatten From String(type=w305, binary string=w303, data includes array or string size? (T)=FALSE) -> (value=w304:T8, error out=w306:errorcluster)  [unwired: 2 in, 1 out]
                n207 = case shown="No Error" w306 {
                  tunnel: w304 -> [w310 _]
                  tunnel: w303 -> [_ w311]
                  frame No Error {
                    n208 = Unbundle By Name(w310) -> ("ref_vel"=w309:dbl, "ref_steer"=w308:dbl)
                    n209 = global write "rio_Global.vi" "Ref_VS"(w309) -> ()
                    n210 = global write "rio_Global.vi" "Ref_str_ang"(w308) -> ()
                  }
                  frame Error {
                    n211 = global read "rio_Global.vi" "CON_INPUT_T"() -> (w313:T9)
                    n212 = Unflatten From String(type=w313, binary string=w311, data includes array or string size? (T)=FALSE) -> (value=w312:T9, error out=w314:errorcluster)  [unwired: 2 in, 1 out]
                    n213 = case shown="No Error" w314 {
                      tunnel: w312 -> [w318 _]
                      frame No Error {
                        n214 = Unbundle By Name(w318) -> ("ref_vel"=w317:dbl, "ref_steer"=w316:dbl)
                        n215 = global write "rio_Global.vi" "Ref_VS"(w317) -> ()
                        n216 = global write "rio_Global.vi" "Ref_str_ang"(w316) -> ()
                      }
                      frame Error {
                      }
                    }
                  }
                }
              }
            }
          }
          frame #2 {
            n217 = local read "Con_time 10"() -> (w321:i32)
            n218 = global read "rio_Global.vi" "C_MCP"() -> (→"C_MCP":dbl)
            n219 = global read "rio_Global.vi" "C_APV"() -> (→"C_APV":dbl)
            n220 = global read "rio_Global.vi" "Ref_VS"() -> (w328:dbl)
            "Ref_VS" <- w328
            n221 = To Double Precision Float(number=w321) -> (double precision float=w320:dbl)
            n222 = Select(t=w328, s="Velocity input", f="Manual Speed") -> (s? t:f=w331:dbl)
            n223 = flat-sequence {
              tunnel: w331 -> [w363]
              tunnel: [w364] -> w333
              frame #0 {
                n224 = global read "rio_Global.vi" "C_VS_CAN"() -> (w367:dbl)
                "VS_CAN" <- w367
                n225 = global read "rio_Global.vi" "Car_name"() -> (w365:string)
                n226 = Subtract(x=w363, y=w367) -> (x-y=w366:dbl)
                n227 = case shown="\"Santafe\", Default" w365 {
                  tunnel: w366 -> [w369 w432]
                  tunnel: [w372 w431] -> w364
                  tunnel: w363 -> [w377 w426]
                  frame "Santafe", Default {
                    w371 = 5.0 ("gain accel")
                    w381 = 12.0 ("y")
                    # "error"
                    # "ref speed"
                    n228 = Less?(x=w369, y=-2.0 ("lower limit")) -> (x < y?=w388:bool)
                    n229 = Subtract(x=w377, y=20.0) -> (x-y=w385:dbl)
                    n230 = In Range and Coerce(upper limit=20.0, x=w369, lower limit=-10.0) -> (coerced(x)=w378:dbl)  [unwired: 1 out]
                    n231 = case shown="True" w388 {
                      tunnel: [w393 w415] -> w387
                      tunnel: w377 -> [w397 w416]
                      tunnel: w369 -> [w399 w407]
                      frame False {
                        n232 = Greater?(x=w399, y=1.0) -> (0:w402:bool)
                        n233 = global read "rio_Global.vi" "PWM Brake"() -> (w406:dbl)
                        n234 = Equal To 0?(x=w397) -> (x = 0?=w396:bool)
                        n235 = Multiply(x=w406, y=0.999) -> (x*y=w404:dbl)
                        n236 = Max & Min(x=w404, y=1000.0) -> (max(x,y)=w400:dbl)  [unwired: 1 out]
                        n237 = Select(t=1000.0, s=w402, f=w400) -> (s? t:f=w394:dbl)
                        n238 = Select(t=2000.0, s=w396, f=w394) -> (s? t:f=w393:dbl)
                      }
                      frame True {
                        w413 = 0.5 ("gain brake")
                        w422 = 10.0 ("y")
                        n239 = Absolute Value(x=w407) -> (abs(x)=w424:dbl)
                        n240 = Add(x=w424, y=w422) -> (x+y=w423:dbl)
                        n241 = Multiply(x=w423, y=w422) -> (x*y=w421:dbl)
                        n242 = Threshold 1D Array(2:w421, 3:dbl[] [10.0, 15.0, 25.0, 50.0, 80.0, 120.0, 170.0, 230.0, 290.0, 350.0, 420.0]) -> (0:w419:dbl)  [unwired: 1 in]
                        n243 = global read "rio_Global.vi" "PWM Brake"() -> (w411:dbl)
                        n244 = Interpolate 1D Array(1:w419, 2:dbl[] [1000.0, 1100.0, 1200.0, 1300.0, 1400.0, 1500.0, 1600.0, 1700.0, 1800.0, 1900.0, 2000.0]) -> (0:w414:dbl)
                        n245 = Decrement(x=w413) -> (x-1=w412:dbl)
                        n246 = Multiply(x=w414, y=w413) -> (x*y=w409:dbl)
                        n247 = Multiply(x=w412, y=w411) -> (x*y=w410:dbl)
                        n248 = Subtract(x=w409, y=w410) -> (x-y=w408:dbl)
                        n249 = Equal To 0?(x=w416) -> (x = 0?=w417:bool)
                        n250 = Select(t=2000.0, s=w417, f=w408) -> (s? t:f=w415:dbl)
                      }
                    }
                    n251 = Multiply(x=w385, y=0.4) -> (x*y=w383:dbl)
                    n252 = Add(x=w383, y=w381) -> (x+y=w382:dbl)
                    n253 = In Range and Coerce(upper limit=35.0, x=w382, lower limit=w381) -> (coerced(x)=w379:dbl)  [unwired: 1 out]
                    n254 = Multiply(x=w378, y=w379) -> (x*y=w368:dbl)
                    n255 = Multiply(x=w368, y=w371) -> (x*y=w374:dbl)
                    n256 = Decrement(x=w371) -> (x-1=w370:dbl)
                    n257 = feedback-in #4(w368) -> ()
                    n258 = feedback #4(0.0) -> (w375:dbl)
                    n259 = Multiply(x=w370, y=w375) -> (x*y=w373:dbl)
                    n260 = Subtract(x=w374, y=w373) -> (x-y=w372:dbl)
                    n261 = disable-structure shown="Enabled" {
                      disable-tunnel: w387 -> [w392 _]
                      frame Enabled {
                        n262 = global write "rio_Global.vi" "PWM Brake"(w392) -> ()
                      }
                      frame Disabled {
                      }
                    }
                  }
                  frame "Avante" {
                    w438 = dbl[] [20.0, 25.0, 5.0]  # V_PID_gain_avnate
                    n263 = Equal To 0?(x=w426) -> (x = 0?=w427:bool)
                    n264 = In Range and Coerce(upper limit=20.0, x=w432, lower limit=-999.0) -> (coerced(x)=w434:dbl)  [unwired: 1 out]
                    n265 = Select(t=1900.0, s=w427, f=1000.0) -> (s? t:f=w428:dbl)
                    n266 = feedback #5(w434) -> (w436:dbl)
                    n267 = feedback-in #5(w434) -> ()
                    n268 = Absolute Value(x=w434) -> (abs(x)=w442:dbl)
                    n269 = Multiply(x=w434, y=0.01) -> (x*y=w452:dbl)
                    n270 = global write "rio_Global.vi" "PWM Brake"(w428) -> ()
                    n271 = Subtract(x=w434, y=w436) -> (x-y=w435:dbl)
                    n272 = Greater?(x=w442, y=1.0) -> (0:w439:bool)
                    n273 = feedback #6(0.0) -> (w451:dbl)
                    n274 = Multiply(x=w451, y=0.95) -> (x*y=w445:dbl)
                    n275 = Add(x=w445, y=w452) -> (x+y=w446:dbl)
                    n276 = feedback-in #6(w446) -> ()
                    n277 = Select(t=w434, s=w439, f=0.0) -> (s? t:f=w449:dbl)
                    n278 = Divide(x=w435, y=0.01) -> (x/y=w433:dbl)
                    n279 = Build Array(w449, w446, w433) -> (w448:dbl[])
                    n280 = Multiply(x=w438, y=w448) -> (x*y=w447:dbl[])
                    n281 = Add Array Elements(numeric array=w447) -> (sum=w431:dbl)
                  }
                }
              }
            }
            n282 = Multiply(x=w320, y=0.001) -> (x*y=w322:dbl)
            n283 = Max & Min(x=w322, y=0.005) -> (max(x,y)=→"con_dt":dbl)  [unwired: 1 out]
            n284 = Not Equal To 0?(x=w331) -> (x != 0?=w326:bool)
            n285 = global read "rio_Global.vi" "C_Brake"() -> (w330:bool)
            n286 = local read "T out"() -> (w335:i32)
            n287 = local read "T init"() -> (w336:i32)
            n288 = Greater Or Equal?(x=w336, y=w335) -> (x >= y?=w332:bool)
            n289 = Not(x=w330) -> (.not. x?=w329:bool)
            n290 = Compound Arithmetic op=AND(w332, w329, w326) -> (w334:bool)
            n291 = case shown="True" w334 {
              tunnel: [1000.0 ("Numeric") w355] -> w337
              tunnel: w333 -> [_ w357]
              tunnel: w335 -> [w341 _]
              tunnel: [_ TRUE] -> w338
              frame False {
                n292 = local read "T init"() -> (w342:i32)
                n293 = Less Or Equal?(x=w342, y=w341) -> (x <= y?=w343:bool)
                n294 = case shown="False" w343 {
                  tunnel: w341 -> [_ w346]
                  frame False {
                    n295 = local write "T init"(1 ("T init")) -> ()
                  }
                  frame True {
                    n296 = local read "T init"() -> (w349:i32)
                    n297 = Increment(x=w349) -> (x+1=w348:i32)
                    n298 = Max & Min(x=w348, y=w346) -> (min(x,y)=w347:i32)  [unwired: 1 out]
                    n299 = local write "T init"(w347) -> ()
                  }
                }
              }
              frame True {
                n300 = To Long Integer(number=w357) -> (32bit integer=w359:i32)
                n301 = Multiply(x=10.0, y=w357) -> (x*y=w354:dbl)
                n302 = Add(x=w359, y=20) -> (x+y=w361:i32)
                "T out" <- w361
                n303 = Add(x=w354, y=1000.0 ("PWM GAS")) -> (x+y=w352:dbl)
                n304 = Increment(x=w361) -> (x+1=→"T init":i32)
                n305 = In Range and Coerce(upper limit=1600.0, x=w352, lower limit=1000.0 ("x")) -> (coerced(x)=w355:dbl)  [unwired: 1 out]
              }
            }
            "PWM GAS" <- w337
            n306 = global write "rio_Global.vi" "Solenoid"(w338) -> ()
            n307 = global write "rio_Global.vi" "PWM GAS"(w337) -> ()
          }
          frame #3 {
            n308 = disable-structure shown="Enabled" {
              disable-tunnel: [w562 "Dial"] -> w456
              frame Disabled {
                n309 = global read "rio_Global.vi" "Ref_str_ang"() -> (w562:dbl)
              }
              frame Enabled {
              }
            }
            n310 = disable-structure shown="Enabled" {
              disable-tunnel: [_ w504] -> w455
              disable-tunnel: w456 -> [_ w497]
              frame Disabled {
                w485 = 0.6000000000000001 ("y")
                n311 = Absolute Value() -> (x=w460:dbl, abs(x)=w479:dbl)
                n312 = Not A Number/Path/Refnum?(number/path/refnum=w460) -> (NaN/Path/Refnum?=w488:bool)
                n313 = Select(t=0.0, s=w488, f=w460) -> (s? t:f=w487:dbl)
                n314 = Multiply(x=w479, y=-0.02) -> (x*y=w477:dbl)
                n315 = Add(x=w477, y=1.1) -> (x+y=w475:dbl)
                n316 = In Range and Coerce(upper limit=0.22, x=w475, lower limit=0.08) -> (coerced(x)=w472:dbl)  [unwired: 1 out]
                n317 = global read "rio_Global.vi" "C_mdps str_ang"() -> (w464:dbl)
                n318 = Negate(x=w472) -> (-x=w470:dbl)
                n319 = Bundle By Name(cluster=T7 {"proportional gain (Kc)"=-0.1, "integral time (Ti, min)"=0.0, "derivative time (Td, min)"=0.0} ("PID gains"), "proportional gain (Kc)"=w470) -> (w469:T7)
                n320 = Not A Number/Path/Refnum?(number/path/refnum=w464) -> (NaN/Path/Refnum?=w492:bool)
                n321 = Select(t=0.0, s=w492, f=w464) -> (s? t:f=w490:dbl)
                n322 = call-poly <vilib>:"PID.vi"("output range"=cluster{"output high":dbl, "output low":dbl} {"output high"=5.0, "output low"=-5.0}, "dt (s)"=-1.0, "PID gains"=w469, "process variable"=w490, "setpoint"=w487) -> ("output"=w486:dbl)  [unwired: 5 in, 1 out]
                n323 = Decrement(x=w485) -> (x-1=w484:dbl)
                n324 = Multiply(x=w486, y=w485) -> (x*y=w481:dbl)
                n325 = global read "rio_Global.vi" "C_mdps torque"() -> (w462:dbl)
                n326 = feedback #7(0.0) -> (w483:dbl)
                n327 = Multiply(x=w484, y=w483) -> (x*y=w482:dbl)
                n328 = Subtract(x=w481, y=w482) -> (x-y=w466:dbl)
                n329 = Not A Number/Path/Refnum?(number/path/refnum=w466) -> (NaN/Path/Refnum?=w468:bool)
                n330 = Select(t=0.0, s=w468, f=w466) -> (s? t:f=w465:dbl)
                n331 = feedback-in #7(w465) -> ()
                n332 = Multiply(x=-0.05 ("x 5"), y=w462) -> (x*y=w461:dbl)
                n333 = Multiply(x=0.1 ("x 2"), y=w465) -> (x*y=w493:dbl)
                n334 = Add(x=w493, y=w461) -> ()  [unwired: 1 out]
              }
              frame Enabled {
                n335 = global read "rio_Global.vi" "C_mdps str_ang"() -> (w499:dbl)
                n336 = disable-structure shown="Enabled" {
                  disable-tunnel: [w532 w541] -> w498
                  disable-tunnel: w499 -> [w531 w541]
                  frame Enabled {
                    n337 = flat-sequence {
                      tunnel: w531 -> [w540]
                      tunnel: [w534] -> w532
                      frame #0 {
                        n338 = Multiply(x=w540, y="lpf gain 2") -> (x*y=w538:dbl)
                        n339 = Decrement(x="lpf gain 2") -> (x-1=w539:dbl)
                        n340 = feedback #8(0.0) -> (w536:dbl)
                        n341 = Multiply(x=w539, y=w536) -> (x*y=w537:dbl)
                        n342 = Subtract(x=w538, y=w537) -> (x-y=w534:dbl)
                        n343 = feedback-in #8(w534) -> ()
                      }
                    }
                  }
                  frame Disabled {
                  }
                }
                n344 = local read "con_dt"() -> (w502:dbl)
                n345 = Multiply(x=w502, y=4.0) -> (x*y=w501:dbl)
                n346 = Add(x=w498, y=w497) -> (x+y=w503:dbl)
                n347 = flat-sequence {
                  tunnel: w503 -> [w543]
                  tunnel: [w542] -> w514
                  frame #0 {
                    n348 = disable-structure shown="Enabled" {
                      disable-tunnel: w543 -> [w545 w550]
                      disable-tunnel: [w544 w550] -> w542
                      frame Enabled {
                        n349 = Absolute Value(x=w545) -> (abs(x)=w549:dbl)
                        n350 = Greater?(x=w549, y=0.4) -> (0:w547:bool)
                        n351 = Select(t=w545, s=w547, f=0.0) -> (s? t:f=w544:dbl)
                      }
                      frame Disabled {
                      }
                    }
                    "Waveform Chart 2" <- w542
                  }
                }
                n352 = call <vilib>:"Derivative x(t) PtByPt.vi"("initialize"=FALSE, "dt"=w501, "initial condition"=0.0, "x"=w498) -> ("dx/dt"=w507:dbl)  [unwired: 1 out]
                n353 = Multiply(x="d gain", y=w507) -> (x*y=w506:dbl)
                n354 = local read "con_dt"() -> (w517:dbl)
                n355 = Multiply(x="p gain", y=w514) -> (x*y=w505:dbl)
                n356 = local read "p gain"() -> (w520:dbl)
                n357 = Reciprocal(x=w520) -> (1/x=w509:dbl)
                n358 = feedback #9(0.0) -> (w516:dbl)
                n359 = Add(x=w514, y=w516) -> (x+y=w518:dbl)
                n360 = call <vilib>:"Integral x(t) PtByPt.vi"("initialize"=FALSE, "dt"=w517, "initial condition"=0.0, "x"=w518) -> ("integral x(t)"=w528:dbl)  [unwired: 1 out]
                n361 = Compound Arithmetic op=MULTIPLY(w528, "i gain", 0.01 ("x")) -> (w515:dbl)
                n362 = Compound Arithmetic op=ADD(w506, w505, w515) -> (w512:dbl)
                n363 = In Range and Coerce(upper limit=0.55, x=w512, lower limit=-0.55) -> (coerced(x)=w511:dbl)  [unwired: 1 out]
                n364 = Subtract(x=w511, y=w512) -> (x-y=w510:dbl)
                n365 = disable-structure shown="Enabled" {
                  disable-tunnel: w511 -> [w552 w561]
                  disable-tunnel: [w551 w561] -> w504
                  frame Enabled {
                    n366 = flat-sequence {
                      tunnel: w552 -> [w560]
                      tunnel: [w554] -> w551
                      frame #0 {
                        n367 = Multiply(x=w560, y="lpf gain") -> (x*y=w558:dbl)
                        n368 = Decrement(x="lpf gain") -> (x-1=w559:dbl)
                        n369 = feedback #10(0.0) -> (w556:dbl)
                        n370 = Multiply(x=w559, y=w556) -> (x*y=w557:dbl)
                        n371 = Subtract(x=w558, y=w557) -> (x-y=w554:dbl)
                        n372 = feedback-in #10(w554) -> ()
                      }
                    }
                  }
                  frame Disabled {
                  }
                }
                n373 = Multiply(x=w510, y=w509) -> (x*y=w519:dbl)
                n374 = feedback-in #9(w519) -> ()
              }
            }
            n375 = Select(t=w455, s="Steer input", f="Manual Steering torque") -> (s? t:f=w457:dbl)
            "Waveform Chart 3" <- w457
            n376 = global write "rio_Global.vi" "steering torque"(w457) -> ()
          }
          frame #4 {
            n377 = Get Date/Time In Seconds() -> (seconds since 1Jan1904=w569:timestamp)
            n378 = global read "rio_Global.vi" "LCM_CON_T 2"() -> (w578:T10)
            n379 = To Double Precision Float(number=w569) -> (double precision float=w568:dbl)
            n380 = Unbundle By Name(w578) -> ("hash"=w579:i64)
            n381 = Multiply(x=w568, y=1000000.0) -> (x*y=w572:dbl)
            n382 = To Quad Integer(1:w572) -> (0:w570:i64)
            n383 = call "hash.vi"("input"=w579) -> ("output"=w577:i64)  [unwired: 10 in]
            n384 = String To IP(1:"192.168.100.200") -> (0:w565:u32)
            n385 = global read "rio_Global.vi" "Auto"() -> (w564:bool)
            n386 = Bundle By Name(cluster=w578, "hash"=w577, "sys time"=w570, "Auto"=w564, "Run"=w564, "net address"=w565) -> (w567:T10)
            n387 = Flatten To String(anything=w567, prepend array or string size? (T)=FALSE) -> (data string=w574:string)  [unwired: 2 in, 2 out]
            n388 = global read "rio_Global.vi" "LCM"() -> (w576:T4)
            n389 = call "LCM_send.vi"("DATA"=w574, "ID"="CON_T", "LCM"=w576) -> ()  [unwired: 7 in, 2 out]
          }
        }
      }
    }
  }
  n390 = flat-sequence {
    tunnel: [dbl[] [0.0, 0.0, 0.0, 0.0, 0.0] ("pos(i)")] -> w1
    tunnel: w1 -> [w588]
    frame #0 {
      w582 = FALSE ("get heading")
      w583 = u64 1
      w580 = 0.0 ("dh_hat")
      n391 = local write "GPS init"(w582) -> ()
      n392 = call "getecefdcmref.vi"("map name"="map name") -> ("XYZ"=→"ecef ref":dbl[])  [unwired: 10 in, 4 out]
      "map" <- "map name"
      "vgain" <- 1.0 ("initH")
      "vcount" <- w583
      "hbias" <- w580
      "hcount" <- w583
      "get heading" <- w582
      "get position" <- w582
      "heading error" <- w580
      "h_gps" <- w580
      "rt" <- w580
      "pos error" <- w580
      "POS init" <- TRUE ("POS init")
    }
    frame #1 {
      (unwired) FALSE
      n393 = while {
        shift-right: [w665] -> _
        shift-left: w588 -> [w666]
        stop <- FALSE stop-if-true
        n394 = flat-sequence {
          tunnel: [w698] -> w669
          tunnel: w666 -> [w698]
          tunnel: w669 -> [w701]
          tunnel: [w700] -> w668
          tunnel: [w700] -> w667
          tunnel: [w1115] -> w665
          tunnel: w668 -> [w1116]
          tunnel: w667 -> [w1115]
          frame #0 {
            n395 = global read "rio_Global.vi" "C_ts"() -> (→"dt":dbl)
            n396 = global read "rio_Global.vi" "C_WHL_SPD_RR"() -> (w684:dbl)
            n397 = global read "rio_Global.vi" "C_WHL_SPD_RL"() -> (w683:dbl)
            n398 = Wait Until Next ms Multiple(millisecond multiple=u32 10) -> (millisecond timer value=w696:u32)
            n399 = feedback #11(w696) -> (w695:u32)
            n400 = feedback-in #11(w696) -> ()
            n401 = Subtract(x=w696, y=w695) -> (x-y=w694:u32)
            n402 = Subtract(x=w684, y=w683) -> (x-y=w691:dbl)
            n403 = global read "rio_Global.vi" "overall width"() -> (w674:dbl)
            n404 = To Long Integer(number=w694) -> (32bit integer=→"Pos_time 10":i32)
            n405 = Divide(x=w691, y=3.6) -> (x/y=w689:dbl)
            n406 = Divide(x=w689, y=w674) -> (x/y=w688:dbl)
            n407 = global read "rio_Global.vi" "C_VS_CAN"() -> (w676:dbl)
            n408 = global read "rio_Global.vi" "C_yaw_rate"() -> (w673:dbl)
            n409 = Multiply(x=w688, y=180.0) -> (x*y=w686:dbl)
            n410 = Sign(1:w676) -> (0:w675:dbl)
            n411 = Divide(x=w686, y=3.141592653589793) -> (x/y=w680:dbl)
            n412 = Compound Arithmetic op=MULTIPLY(w680, 1.2144 ("scale"), w675) -> (w678:dbl)
            n413 = Multiply(x=w673, y=1.0) -> (x*y=w672:dbl)
            n414 = Select(t=w678, s=FALSE, f=w672) -> (s? t:f=→"C_yaw_rate":dbl)
            n415 = Build Array(w678, w672) -> (w677:dbl[])
            n416 = call "Convert to Dynamic Data"("Array"=w677) -> ()  [unwired: 3 in, 1 out]
          }
          frame #1 {
            n417 = flat-sequence {
              tunnel: w701 -> [w708]
              tunnel: [w708] -> w699
              tunnel: [w831] -> w700
              tunnel: w699 -> [w832]
              frame #0 {
                n418 = disable-structure shown="Enabled" {
                  disable-tunnel: [w728 w729] -> w703
                  disable-tunnel: [w709 w730] -> w702
                  frame Disabled {
                    n419 = global read "rio_Global.vi" "gps_pos 1"() -> (w725:dbl[])
                    n420 = global read "rio_Global.vi" "gps_pos 2"() -> (w712:dbl[])
                    n421 = Add(x=w725, y=w712) -> (x+y=w727:dbl[])
                    n422 = Index Array(array=w725, index #1=0 ("index")) -> (element #1=w724:dbl, element #2=w723:dbl)  [unwired: 1 in]
                    n423 = Index Array(array=w712, index #1=0 ("index")) -> (element #1=w713:dbl, element #2=w714:dbl)  [unwired: 1 in]
                    n424 = feedback #12(w724) -> (w722:dbl)
                    n425 = feedback-in #12(w724) -> ()
                    n426 = feedback #13(w713) -> (w715:dbl)
                    n427 = feedback-in #13(w713) -> ()
                    n428 = Not Equal To 0?(x=w714) -> (x != 0?=w717:bool)
                    n429 = Not Equal?(x=w724, y=w722) -> (x != y?=w721:bool)
                    n430 = Not Equal?(x=w713, y=w715) -> (x != y?=w716:bool)
                    n431 = Not Equal To 0?(x=w723) -> (x != 0?=w720:bool)
                    n432 = And(x=w721, y=w720) -> (x .and. y?=w710:bool)
                    n433 = And(x=w716, y=w717) -> (x .and. y?=w711:bool)
                    n434 = And(x=w710, y=w711) -> (x .and. y?=w728:bool)
                    n435 = Multiply(x=w727, y=0.5) -> (x*y=w709:dbl[])
                  }
                  frame Enabled {
                    n436 = global read "rio_Global.vi" "gps_pos 1"() -> (w730:dbl[])
                    n437 = Index Array(array=w730, index #1=0 ("index")) -> (element #1=w736:dbl, element #2=w735:dbl)  [unwired: 1 in]
                    n438 = feedback #14(w736) -> (w734:dbl)
                    n439 = feedback-in #14(w736) -> ()
                    n440 = Not Equal?(x=w736, y=w734) -> (x != y?=w733:bool)
                    n441 = Not Equal To 0?(x=w735) -> (x != 0?=w732:bool)
                    n442 = And(x=w733, y=w732) -> (x .and. y?=w729:bool)
                  }
                }
                "pos_gps" <- w702
                n443 = disable-structure shown="Enabled" {
                  disable-tunnel: [w782 w813] -> w707
                  disable-tunnel: [w781 w792] -> w706
                  disable-tunnel: [w753 w803] -> w705
                  disable-tunnel: [w741 w798] -> w704
                  frame Disabled {
                    n444 = global read "rio_Global.vi" "gps_vel 1"() -> (w780:dbl[])
                    n445 = global read "rio_Global.vi" "gps_vel 2"() -> (w759:dbl[])
                    n446 = Index Array(array=w780, index #1=0 ("index"), index #2=1 ("index"), index #3=4 ("index"), index #4=2 ("index")) -> (element #1=w771:dbl, element #2=w776:dbl, element #3=w773:dbl, element #4=w745:dbl)
                    n447 = Index Array(array=w759, index #1=0 ("index"), index #2=1 ("index"), index #3=4 ("index"), index #4=2 ("index")) -> (element #1=w768:dbl, element #2=w763:dbl, element #3=w766:dbl, element #4=w744:dbl)
                    n448 = global read "rio_Global.vi" "C_VS_CAN"() -> (w738:dbl)
                    n449 = global read "rio_Global.vi" "C_VS_CAN"() -> (w785:dbl)
                    n450 = Add(x=w745, y=w744) -> (x+y=w743:dbl)
                    n451 = call "angleconv.vi"("deg"=w773) -> ("rad"=w756:dbl)  [unwired: 9 in, 1 out]
                    n452 = call "angleconv.vi"("deg"=w766) -> ("rad"=w755:dbl)  [unwired: 9 in, 1 out]
                    n453 = Not Equal To 0?(x=w763) -> (x != 0?=w764:bool)
                    n454 = feedback #15(0.0 ("Real Matrix Element")) -> (w770:dbl)
                    n455 = feedback-in #15(w771) -> ()
                    n456 = feedback #16(0.0 ("Real Matrix Element")) -> (w769:dbl)
                    n457 = feedback-in #16(w768) -> ()
                    n458 = Not Equal?(x=w771, y=w770) -> (x != y?=w777:bool)
                    n459 = Not Equal?(x=w768, y=w769) -> (x != y?=w762:bool)
                    n460 = Greater Or Equal To 0?(x=w785) -> (x >= 0?=w786:bool)
                    n461 = Not Equal To 0?(x=w776) -> (x != 0?=w775:bool)
                    n462 = Absolute Value(x=w738) -> (abs(x)=w737:dbl)
                    n463 = Multiply(x=w743, y=0.5) -> (x*y=w752:dbl)
                    n464 = call "headingweightsum.vi"("a"=0.5, "h1"=w755, "h2"=w756) -> ("a*h2+(1-a)*h1"=w784:dbl)  [unwired: 8 in]
                    n465 = And(x=w777, y=w775) -> (x .and. y?=w758:bool)
                    n466 = And(x=w762, y=w764) -> (x .and. y?=w757:bool)
                    n467 = Divide(x=w752, y=w737) -> (x/y=w753:dbl)
                    n468 = Select(t=0.0, s=w786, f=3.141592653589793) -> (s? t:f=w783:dbl)
                    n469 = Decrement(x=w753) -> (x-1=w749:dbl)
                    n470 = call "headingoperater.vi"("h1"=w783, "h2"=w784) -> ("h2-h1"=w782:dbl)  [unwired: 8 in, 1 out]
                    n471 = And(x=w758, y=w757) -> (x .and. y?=w781:bool)
                    n472 = Absolute Value(x=w749) -> (abs(x)=w750:dbl)
                    n473 = Greater?(x=w737, y=15.0) -> (0:w739:bool)
                    n474 = Less?(x=w750, y=0.05) -> (x < y?=w742:bool)
                    n475 = Compound Arithmetic op=AND(w739, w742, w781) -> (w741:bool)
                  }
                  frame Enabled {
                    n476 = global read "rio_Global.vi" "gps_vel 1"() -> (w812:dbl[])
                    n477 = global read "rio_Global.vi" "C_VS_CAN"() -> (w796:dbl)
                    n478 = global read "rio_Global.vi" "C_VS_CAN"() -> (w815:dbl)
                    n479 = Index Array(array=w812, index #1=0 ("index"), index #2=1 ("index"), index #3=4 ("index"), index #4=2 ("index")) -> (element #1=w791:dbl, element #2=w808:dbl, element #3=w805:dbl, element #4=w794:dbl)
                    n480 = Greater Or Equal To 0?(x=w815) -> (x >= 0?=w816:bool)
                    n481 = Absolute Value(x=w796) -> (abs(x)=w795:dbl)
                    n482 = feedback #17(w791) -> (w804:dbl)
                    n483 = feedback-in #17(w791) -> ()
                    n484 = Divide(x=w794, y=w795) -> (x/y=w803:dbl)
                    n485 = call "angleconv.vi"("deg"=w805) -> ("rad"=w793:dbl)  [unwired: 9 in, 1 out]
                    n486 = Select(t=0.0, s=w816, f=3.141592653589793) -> (s? t:f=w814:dbl)
                    n487 = Not Equal?(x=w791, y=w804) -> (x != y?=w809:bool)
                    n488 = Decrement(x=w803) -> (x-1=w800:dbl)
                    n489 = Not Equal To 0?(x=w808) -> (x != 0?=w807:bool)
                    n490 = call "headingoperater.vi"("h1"=w814, "h2"=w793) -> ("h2-h1"=w813:dbl)  [unwired: 8 in, 1 out]
                    n491 = And(x=w809, y=w807) -> (x .and. y?=w792:bool)
                    n492 = Absolute Value(x=w800) -> (abs(x)=w801:dbl)
                    n493 = Greater?(x=w795, y=15.0) -> (0:w789:bool)
                    n494 = Less?(x=w801, y=0.05) -> (x < y?=w790:bool)
                    n495 = Compound Arithmetic op=AND(w792, w790, w789) -> (w798:bool)
                  }
                }
                n496 = local write "get position"(w703) -> ()
                n497 = local write "h_gps"(w707) -> ()
                n498 = case shown="True" w704 {
                  tunnel: w705 -> [_ w826]
                  frame False {
                  }
                  frame True {
                    w820 = u64 18446744073709551615
                    n499 = local read "vcount"() -> (w823:u64)
                    n500 = local read "vgain"() -> (w828:dbl)
                    n501 = Increment(x=w823) -> (x+1=w822:u64)
                    n502 = Multiply(x=w828, y=w823) -> (x*y=w827:dbl)
                    n503 = Not Equal?(x=w823, y=w820) -> (x != y?=w821:bool)
                    n504 = Add(x=w826, y=w827) -> (x+y=w825:dbl)
                    n505 = Select(t=w822, s=w821, f=w820) -> (s? t:f=w819:u64)
                    n506 = Divide(x=w825, y=w819) -> (x/y=w824:dbl)
                    n507 = local write "vcount"(w819) -> ()
                    n508 = local write "vgain"(w824) -> ()
                  }
                }
                n509 = local write "get heading"(w706) -> ()
              }
              frame #1 {
                n510 = local read "dt"() -> (w830:dbl)
                n511 = Greater Than 0?(x=w830) -> (x > 0?=w829:bool)
                n512 = case shown="True" w829 {
                  tunnel: w832 -> [w833 w836]
                  tunnel: [w833 w835] -> w831
                  frame False {
                  }
                  frame True {
                    n513 = flat-sequence {
                      tunnel: w836 -> [w871]
                      tunnel: [w849] -> w834
                      tunnel: [w899] -> w835
                      tunnel: w834 -> [w898]
                      frame #0 {
                        n514 = global read "rio_Global.vi" "C_VS_CAN"() -> (w839:dbl)
                        n515 = local read "C_yaw_rate"() -> (w837:dbl)
                        n516 = Equal To 0?(x=w839) -> (x = 0?=w841:bool)
                        n517 = case shown="True" w841 {
                          tunnel: [w873 _] -> w840
                          tunnel: w837 -> [w872 w877]
                          frame False {
                            n518 = local read "hbias"() -> (w876:dbl)
                            n519 = Subtract(x=w872, y=w876) -> (x-y=w874:dbl)
                            n520 = Negate(x=w874) -> (-x=w875:dbl)
                            n521 = call "angleconv.vi"("deg"=w875) -> ("rad"=w873:dbl)  [unwired: 9 in, 1 out]
                          }
                          frame True {
                            w880 = u64 18446744073709551615
                            n522 = local read "hcount"() -> (w883:u64)
                            n523 = local read "hbias"() -> (w886:dbl)
                            n524 = Increment(x=w883) -> (x+1=w882:u64)
                            n525 = Not Equal?(x=w883, y=w880) -> (x != y?=w881:bool)
                            n526 = Multiply(x=w886, y=w883) -> (x*y=w885:dbl)
                            n527 = Add(x=w877, y=w885) -> (x+y=w884:dbl)
                            n528 = Select(t=w882, s=w881, f=w880) -> (s? t:f=w879:u64)
                            n529 = local write "hcount"(w879) -> ()
                            n530 = Divide(x=w884, y=w879) -> (x/y=w878:dbl)
                            n531 = local write "hbias"(w878) -> ()
                          }
                        }
                        n532 = global read "rio_Global.vi" "C_VS_CAN"() -> (w838:dbl)
                        n533 = local read "vgain"() -> (w844:dbl)
                        n534 = Multiply(x=w838, y=w844) -> (x*y=w843:dbl)
                        n535 = Divide(x=w843, y=3.6) -> (x/y=w842:dbl)
                        n536 = Index Array(array=w871, index #1=0 ("index"), index #2=3 ("index"), index #3=1 ("index"), index #4=3 ("index")) -> (element #1=w865:dbl, element #2=w863:dbl, element #3=w859:dbl, element #4=w854:dbl)
                        n537 = local read "dt"() -> (w868:dbl)
                        n538 = local read "dt"() -> (w852:dbl)
                        n539 = Multiply(x=w842, y=w868) -> (x*y=w864:dbl)
                        n540 = Multiply(x=w852, y=w840) -> (x*y=w845:dbl)
                        n541 = Cosine(x=w863) -> (cos(x)=w869:dbl)
                        n542 = Sine(x=w863) -> (sin(x)=w862:dbl)
                        n543 = Multiply(x=w869, y=w864) -> (x*y=w866:dbl)
                        n544 = Multiply(x=w864, y=w862) -> (x*y=w861:dbl)
                        n545 = local write "rt"(w845) -> ()
                        n546 = Add(x=w865, y=w866) -> (x+y=w858:dbl)
                        n547 = Add(x=w861, y=w859) -> (x+y=w857:dbl)
                        n548 = call "headingoperater.vi"("h1"=w845, "h2"=w854) -> ("h2+h1"=w853:dbl)  [unwired: 8 in, 1 out]
                        n549 = Build Array(w858, w857, w842, w853, w840) -> (w849:dbl[])
                        n550 = Index Array(array=w849, index=3) -> (element=w848:dbl)
                        n551 = local read "h_gps"() -> (w847:dbl)
                        n552 = call "headingoperater.vi"("h1"=w848, "h2"=w847) -> ("h2-h1"=w851:dbl)  [unwired: 8 in, 1 out]
                        n553 = Absolute Value(x=w851) -> (abs(x)=w846:dbl)
                        n554 = local write "heading error"(w846) -> ()
                      }
                      frame #1 {
                        n555 = local read "get heading"() -> (w906:bool)
                        n556 = local read "get position"() -> (w905:bool)
                        n557 = local read "POS init"() -> (w891:bool)
                        n558 = case shown="False" w891 {
                          tunnel: w906 -> [w909 w916]
                          tunnel: w905 -> [w913 w915]
                          tunnel: [w907 w914] -> w901
                          frame False {
                            n559 = local read "heading error"() -> (w910:dbl)
                            n560 = Less?(x=w910, y=0.05) -> (x < y?=w911:bool)
                            n561 = And(x=w909, y=w911) -> (x .and. y?=w908:bool)
                            n562 = Or(x=w908, y=w913) -> (x .or. y?=w907:bool)
                          }
                          frame True {
                            n563 = disable-structure shown="Enabled" {
                              disable-tunnel: w916 -> [w919 w921]
                              disable-tunnel: w915 -> [w918 w920]
                              disable-tunnel: [w917 w922] -> w914
                              frame Disabled {
                                n564 = And(x=w919, y=w918) -> (x .and. y?=w917:bool)
                              }
                              frame Enabled {
                                n565 = Or(x=w921, y=w920) -> (x .or. y?=w922:bool)
                              }
                            }
                          }
                        }
                        n566 = global read "rio_Global.vi" "C_VS_CAN"() -> (w904:dbl)
                        n567 = local read "heading error"() -> (w894:dbl)
                        n568 = Absolute Value(x=w904) -> (abs(x)=w903:dbl)
                        n569 = local read "POS init"() -> (w892:bool)
                        n570 = Greater?(x=w903, y=5.0) -> (0:w900:bool)
                        n571 = Less?(x=w894, y=1.0) -> (x < y?=w893:bool)
                        n572 = Or(x=w893, y=w892) -> (x .or. y?=w895:bool)
                        n573 = And(x=w901, y=w900) -> (x .and. y?=w896:bool)
                        n574 = And(x=w896, y=w895) -> (x .and. y?=w889:bool)
                        n575 = Select(t=FALSE, s="GPS init", f=w889) -> (s? t:f=w888:bool)
                        n576 = case shown="True" w888 {
                          tunnel: [w926 w955] -> w899
                          tunnel: w898 -> [w927 w958]
                          frame False {
                            n577 = global read "rio_Global.vi" "C_VS_CAN"() -> (w930:dbl)
                            n578 = local read "POS init"() -> (w929:bool)
                            n579 = Equal To 0?(x=w930) -> (x = 0?=w928:bool)
                            n580 = local read "GPS init"() -> (w923:bool)
                            n581 = And(x=w929, y=w928) -> (x .and. y?=w925:bool)
                            n582 = Or(x=w925, y=w923) -> (x .or. y?=w924:bool)
                            n583 = case shown="True" w924 {
                              tunnel: w927 -> [w931 w932]
                              tunnel: [w931 w934] -> w926
                              tunnel: w923 -> [_ w933]
                              frame False {
                              }
                              frame True {
                                n584 = case shown="True" w933 {
                                tunnel: [w945 w954] -> w934
                                tunnel: w932 -> [w940 w948]
                                frame True {
                                n585 = Index Array(array=w940, index #1=2 ("index")) -> (element #2=w935:dbl, element #3=w938:dbl)  [unwired: 2 in, 1 out]
                                n586 = local read "pos_gps"() -> (w941:dbl[])
                                n587 = local write "GPS init"(FALSE ("GPS init")) -> ()
                                n588 = Index Array(array=w941, index #1=2 ("index")) -> (element #1=w943:dbl, element #2=w942:dbl)  [unwired: 1 in]
                                n589 = local read "h_gps"() -> (w936:dbl)
                                n590 = Build Array(w943, w942, w935, w936, w938) -> (w945:dbl[])
                                }
                                frame False {
                                w947 = 0.0 ("element")
                                n591 = Index Array(array=w948, index=3) -> (element=w946:dbl)
                                n592 = local read "pos_gps"() -> (w950:dbl[])
                                n593 = Index Array(array=w950, index #1=2 ("index")) -> (element #1=w952:dbl, element #2=w951:dbl)  [unwired: 1 in]
                                n594 = Build Array(w952, w951, w947, w946, w947) -> (w954:dbl[])
                                }
                                }
                              }
                            }
                          }
                          frame True {
                            n595 = flat-sequence {
                              tunnel: w958 -> [w959]
                              tunnel: [w959] -> w957
                              tunnel: w957 -> [w1000]
                              tunnel: [w1000] -> w956
                              tunnel: w956 -> [w1027]
                              tunnel: [w1031] -> w955
                              frame #0 {
                                w968 = 0.0 ("element")
                                w972 = 0.0 ("element")
                                w974 = 0.0 ("element")
                                w976 = 0.0 ("element")
                                w978 = 0.0 ("element")
                                n596 = Index Array(array=w959, index #1=3 ("index"), index #2=2 ("index"), index #3=3 ("index"), index #4=2 ("index")) -> (element #1=w988:dbl, element #2=w990:dbl, element #3=w993:dbl, element #4=w982:dbl)
                                n597 = Negate(x=w990) -> (-x=w989:dbl)
                                n598 = Sine & Cosine(0:w993) -> (1:w985:dbl, 2:w983:dbl)
                                n599 = Multiply(x=w989, y=w985) -> (x*y=w986:dbl)
                                n600 = Multiply(x=w983, y=w982) -> (x*y=w981:dbl)
                                n601 = Cosine(x=w988) -> (cos(x)=w987:dbl)
                                n602 = Build Array(w978, w978, w987, w986, 0.0 ("element")) -> (w980:dbl[])
                                n603 = Build Array(w976, w976, w985, w981, 0.0 ("element")) -> (w979:dbl[])
                                n604 = Build Array(w974, w974, w974, w974, w974) -> (w973:dbl[])
                                n605 = Build Array(w972, w972, w972, w972, 1.0 ("element")) -> (w970:dbl[])
                                n606 = Build Array(w968, w968, w968, w968, w968) -> (w969:dbl[])
                                n607 = Build Array(w980, w979, w973, w970, w969) -> (w966:dbl[][])
                                n608 = call-poly <vilib>:"Array To Matrix.vi"("Real 2D Array"=w966) -> ("Real Matrix"=w964:T11)
                                n609 = global read "rio_Global.vi" "P"() -> (w967:T11)
                                n610 = Transpose Matrix(1:w964) -> (0:w963:T11)
                                n611 = call-poly <vilib>:"Multiply.vi"("Real Matrix B"=w967, "Real Matrix A"=w964) -> ("A * B"=w965:T11)
                                n612 = call-poly <vilib>:"Multiply.vi"("Real Matrix B"=w963, "Real Matrix A"=w965) -> ("A * B"=w962:T11)
                                n613 = global read "rio_Global.vi" "Q"() -> (w961:T11)
                                n614 = call-poly <vilib>:"Add.vi"("Real Matrix B"=w961, "Real Matrix A"=w962) -> ("A + B"=w960:T11)
                                n615 = global write "rio_Global.vi" "Pp"(w960) -> ()
                              }
                              frame #1 {
                                n616 = global read "rio_Global.vi" "Pp"() -> (w1025:T11)
                                n617 = global read "rio_Global.vi" "H"() -> (w1024:T11)
                                n618 = Array Subset(array=w1000, index=0, length=2) -> (w1007:dbl[])
                                n619 = local read "pos_gps"() -> (w1003:dbl[])
                                n620 = call-poly <vilib>:"Multiply.vi"("Real Matrix B"=w1025, "Real Matrix A"=w1024) -> ("A * B"=w1023:T11)
                                n621 = Transpose Matrix(1:w1024) -> (0:w1022:T11)
                                n622 = call-poly <vilib>:"Multiply.vi"("Real Matrix B"=w1022, "Real Matrix A"=w1023) -> ("A * B"=w1021:T11)
                                n623 = Array Subset(array=w1003, index=2, length=2) -> (w1006:dbl[])
                                n624 = Subtract(x=w1006, y=w1007) -> (x-y=w1008:dbl[])
                                n625 = global read "rio_Global.vi" "H"() -> (w1019:T11)
                                n626 = global read "rio_Global.vi" "R"() -> (w1020:T11)
                                n627 = global read "rio_Global.vi" "Pp"() -> (w1018:T11)
                                n628 = call-poly <vilib>:"Add.vi"("Real Matrix B"=w1020, "Real Matrix A"=w1021) -> ("A + B"=w1015:T11)
                                n629 = Square(x=w1008) -> (x^2=w1009:dbl[])
                                n630 = Transpose Matrix(1:w1019) -> (0:w1017:T11)
                                n631 = local read "heading error"() -> (w1012:dbl)
                                n632 = call-poly <vilib>:"Multiply.vi"("Real Matrix B"=w1017, "Real Matrix A"=w1018) -> ("A * B"=w1016:T11)
                                n633 = Add Array Elements(numeric array=w1009) -> (sum=w1010:dbl)
                                n634 = call-poly <vilib>:"Inverse Matrix.vi"("Input Matrix"=w1015) -> ("Inverse Matrix"=w1014:T11)  [unwired: 1 in, 1 out]
                                n635 = call-poly <vilib>:"Multiply.vi"("Real Matrix B"=w1014, "Real Matrix A"=w1016) -> ("A * B"=w1013:T11)
                                n636 = Square Root(x=w1010) -> (sqrt(x)=w999:dbl)
                                n637 = global write "rio_Global.vi" "K"(w1013) -> ()
                                n638 = Less?(x=w999, y=2.5) -> (x < y?=w996:bool)
                                n639 = Less?(x=w1012, y=0.05) -> (x < y?=w997:bool)
                                n640 = And(x=w997, y=w996) -> (x .and. y?=w995:bool)
                                n641 = case shown="True" w995 {
                                frame False {
                                }
                                frame True {
                                n642 = local write "POS init"(FALSE ("Kalman init")) -> ()
                                }
                                }
                              }
                              frame #2 {
                                n643 = disable-structure shown="Enabled" {
                                disable-tunnel: [w1049 w1051] -> w1029
                                disable-tunnel: w1027 -> [_ w1060]
                                frame Disabled {
                                n644 = local read "get position"() -> (w1049:bool)
                                }
                                frame Enabled {
                                n645 = Array Subset(array=w1060, index=0, length=2) -> (w1058:dbl[])
                                n646 = local read "pos_gps"() -> (w1063:dbl[])
                                n647 = Array Subset(array=w1063, index=2, length=2) -> (w1059:dbl[])
                                n648 = disable-structure shown="Enabled" {
                                disable-tunnel: [w1066 TRUE ("Kalman init")] -> w1053
                                frame Disabled {
                                n649 = local read "POS init"() -> (w1066:bool)
                                }
                                frame Enabled {
                                }
                                }
                                n650 = Subtract(x=w1059, y=w1058) -> (x-y=w1057:dbl[])
                                n651 = Square(x=w1057) -> (x^2=w1056:dbl[])
                                n652 = Add Array Elements(numeric array=w1056) -> (sum=w1055:dbl)
                                n653 = Square Root(x=w1055) -> (sqrt(x)=w1050:dbl)
                                n654 = local write "pos error"(w1050) -> ()
                                n655 = Less?(x=w1050, y=3.0) -> (x < y?=w1052:bool)
                                n656 = Or(x=w1053, y=w1052) -> (x .or. y?=w1051:bool)
                                }
                                }
                                n657 = disable-structure shown="Enabled" {
                                disable-tunnel: [w1043 w1044] -> w1030
                                frame Disabled {
                                n658 = local read "get heading"() -> (w1043:bool)
                                }
                                frame Enabled {
                                n659 = local read "heading error"() -> (w1047:dbl)
                                n660 = local read "POS init"() -> (w1045:bool)
                                n661 = Less?(x=w1047, y=0.1) -> (x < y?=w1046:bool)
                                n662 = Or(x=w1046, y=w1045) -> (x .or. y?=w1044:bool)
                                }
                                }
                                n663 = Index Array(array=w1027, index=3) -> (element=w1034:dbl)
                                n664 = global read "rio_Global.vi" "K"() -> (w1042:T11)
                                n665 = global read "rio_Global.vi" "H"() -> (w1041:T11)
                                n666 = global read "rio_Global.vi" "Pp"() -> (w1039:T11)
                                n667 = call-poly <vilib>:"Multiply.vi"("Real Matrix B"=w1041, "Real Matrix A"=w1042) -> ("A * B"=w1040:T11)
                                n668 = global read "rio_Global.vi" "Pp"() -> (w1037:T11)
                                n669 = call-poly <vilib>:"Multiply.vi"("Real Matrix B"=w1039, "Real Matrix A"=w1040) -> ("A * B"=w1038:T11)
                                n670 = call-poly <vilib>:"Subtract.vi"("Real Matrix B"=w1038, "Real Matrix A"=w1037) -> ("A - B"=w1036:T11)
                                n671 = global write "rio_Global.vi" "P"(w1036) -> ()
                                n672 = case shown="True" w1030 {
                                tunnel: w1034 -> [w1092 w1099]
                                tunnel: [w1092 w1094] -> w1028
                                frame False {
                                }
                                frame True {
                                n673 = global read "rio_Global.vi" "K"() -> (w1098:T11)
                                n674 = Index Array(array=w1098, index (row)=3, index (col)=2 ("disabled index (col)")) -> (element=w1095:dbl)
                                n675 = local read "h_gps"() -> (w1093:dbl)
                                n676 = call "headingweightsum2.vi"("a"=w1095, "h2"=w1093, "h1"=w1099) -> ("a*h2+(1-a)*h1"=w1094:dbl)  [unwired: 8 in]
                                }
                                }
                                n677 = case shown="True" w1029 {
                                tunnel: w1027 -> [w1068 w1080]
                                tunnel: [w1068 w1079] -> w1033
                                tunnel: w1028 -> [_ w1069]
                                frame False {
                                }
                                frame True {
                                n678 = disable-structure shown="Enabled" {
                                disable-tunnel: [w1090 w1091] -> w1070
                                disable-tunnel: w1069 -> [_ w1091]
                                frame Disabled {
                                n679 = local read "h_gps"() -> (w1090:dbl)
                                }
                                frame Enabled {
                                }
                                }
                                n680 = local read "pos_gps"() -> (w1074:dbl[])
                                n681 = call-poly <vilib>:"Array To Matrix.vi"("Real 1D Array"=w1080) -> ("Real Matrix (Column Vector)"=w1084:T11)
                                n682 = Array Subset(array=w1074, index=2, length=2) -> (w1075:dbl[])
                                n683 = Build Array (concatenate)(w1075, w1070) -> (w1071:dbl[])
                                n684 = global read "rio_Global.vi" "H"() -> (w1089:T11)
                                n685 = call-poly <vilib>:"Multiply.vi"("Real Matrix B"=w1084, "Real Matrix A"=w1089) -> ("A * B"=w1088:T11)
                                n686 = call-poly <vilib>:"Array To Matrix.vi"("Real 1D Array"=w1071) -> ("Real Matrix (Column Vector)"=w1087:T11)
                                n687 = call-poly <vilib>:"Subtract.vi"("Real Matrix B"=w1088, "Real Matrix A"=w1087) -> ("A - B"=w1085:T11)
                                n688 = global read "rio_Global.vi" "K"() -> (w1086:T11)
                                n689 = call-poly <vilib>:"Multiply.vi"("Real Matrix B"=w1085, "Real Matrix A"=w1086) -> ("A * B"=w1078:T11)
                                n690 = call-poly <vilib>:"Multiply.vi"("Real Matrix A"=w1078, "Real Scalar c"=0.5) -> ("c * A"=w1076:T11)
                                n691 = call-poly <vilib>:"Add.vi"("Real Matrix B"=w1084, "Real Matrix A"=w1076) -> ("A + B"=w1083:T11)
                                n692 = call-poly <vilib>:"Matrix To Array.vi"("Real Matrix"=w1083) -> ("Real 2D Array"=w1082:dbl[][])
                                n693 = Index Array(array=w1082, index (col)=0 ("disabled index (col)")) -> (element=w1079:dbl[])  [unwired: 1 in]
                                }
                                }
                                n694 = Replace Array Subset(array=w1033, new element=w1028, index=3) -> (w1031:dbl[])
                              }
                            }
                          }
                        }
                      }
                    }
                  }
                }
              }
            }
          }
          frame #2 {
            n695 = local read "h_gps"() -> (w1105:dbl)
            n696 = local read "dt"() -> (w1102:dbl)
            n697 = Index Array(array=w1116, index=3) -> (element=w1109:dbl)
            n698 = Array Subset(array=w1116, index=0, length=2) -> (→"pos":dbl[])
            n699 = Greater Than 0?(x=w1102) -> (x > 0?=w1101:bool)
            n700 = call "angleconv.vi"("rad"=w1109) -> ("deg"=→"Heading":dbl)  [unwired: 9 in, 1 out]
            n701 = Greater?(x=1.0, y=w1102) -> (0:w1104:bool)
            n702 = call "headingoperater.vi"("h1"=0.0, "h2"=w1105) -> ("h2+h1"=w1106:dbl)  [unwired: 8 in, 1 out]
            n703 = call "angleconv.vi"("rad"=w1106) -> ("deg"=→"H_GPS":dbl)  [unwired: 9 in, 1 out]
            n704 = Compound Arithmetic op=AND(w1104, w1101) -> (w1100:bool)
            n705 = case shown="True" w1100 {
              tunnel: w1116 -> [_ w1117]
              frame False {
              }
              frame True {
                n706 = flat-sequence {
                  tunnel: w1117 -> [w1141]
                  frame #0 {
                    n707 = Get Date/Time In Seconds() -> (seconds since 1Jan1904=w1132:timestamp)
                    n708 = To Double Precision Float(number=w1132) -> (double precision float=w1126:dbl)
                    n709 = global read "rio_Global.vi" "LCM_POS_T"() -> (w1140:T12)
                    n710 = local read "POS init"() -> (w1122:bool)
                    n711 = Unbundle By Name(w1140) -> ("hash"=w1137:i64)
                    n712 = local read "dt"() -> (w1121:dbl)
                    n713 = Multiply(x=w1126, y=1000000.0) -> (x*y=w1124:dbl)
                    n714 = Array To Cluster(array=w1141) -> (cluster=w1139:T13)
                    n715 = Select(t=0.0, s=w1122, f=w1121) -> (s? t:f=w1119:dbl)
                    n716 = call "hash.vi"("input"=w1137) -> ("output"=w1136:i64)  [unwired: 10 in]
                    n717 = To Quad Integer(1:w1124) -> (0:w1123:i64)
                    n718 = Unbundle(w1139) -> ("Real 2D Array[0]"=w1131:dbl, "Real 2D Array[1]"=w1130:dbl, "Real 2D Array[2]"=w1129:dbl, "Real 2D Array[3]"=w1128:dbl, "Real 2D Array[4]"=w1127:dbl)
                    n719 = Bundle(cluster=w1140, "hash"=w1136, "sys time"=w1123, "dt"=w1119, "x"=w1131, "y"=w1130, "speed"=w1129, "heading"=w1128, "yaw_rate"=w1127) -> (w1118:T12)
                    n720 = Flatten To String(anything=w1118, prepend array or string size? (T)=FALSE) -> (data string=w1134:string)  [unwired: 2 in, 2 out]
                    n721 = global read "rio_Global.vi" "LCM"() -> (w1133:T4)
                    n722 = call "LCM_send.vi"("DATA"=w1134, "ID"="POS_T", "LCM"=w1133) -> ()  [unwired: 7 in, 2 out]
                  }
                }
              }
            }
          }
        }
      }
      n723 = flat-sequence {
        frame #0 {
          n724 = while {
            shift-right: [w595] -> w590
            shift-left: refnum<visa-resource-name> "USB0::0x1546::0x01A8::NI-VISA-1003::1::RAW" ("VISA resource name") -> [w596]
            stop <- w594 continue-if-true
            n725 = VISA Open(VISA resource name=w596) -> (VISA resource name=w595:refnum<visa-resource-name>, error out=w594:errorcluster)  [unwired: 4 in]
          }
          n726 = VISA Clear(VISA resource name=w590) -> (VISA resource name out=w592:refnum<visa-resource-name>)  [unwired: 1 in, 1 out]
          n727 = property class="Instr"(reference=w592, "General Settings:Timeout Value"=u32 10) -> (reference out=→"gps1":refnum<visa-resource-name>)  [unwired: 1 in, 1 out]
        }
        frame #1 {
          n728 = while {
            stop <- FALSE stop-if-true
            n729 = local read "gps1"() -> (w599:refnum<visa-resource-name>)
            n730 = VISA Read(VISA resource name=w599, byte count=u32 100) -> (read buffer=w597:string)  [unwired: 1 in, 3 out]
            n731 = case shown="Default" w597 {
              selector: w597 -> [_ w602]
              frame "" {
                n732 = Wait (ms)(milliseconds to wait=u32 20) -> ()  [unwired: 1 out]
              }
              frame Default {
                n733 = local read "ecef ref"() -> (w603:dbl[])
                n734 = call "nmea.vi"("ecef ref"=w603, "NMEA"=w602) -> ("output"=w605:dbl[], "type"=w604:u32)  [unwired: 8 in]
                n735 = case shown="1" w604 {
                  tunnel: w605 -> [_ w607 w640]
                  frame 0, Default {
                  }
                  frame 1 {
                    n736 = global write "rio_Global.vi" "gps_pos 1"(w607) -> ()
                    n737 = Index Array(array=w607, index=1) -> (element=w609:dbl)
                    n738 = Not Equal To 0?(x=w609) -> (x != 0?=w606:bool)
                    n739 = case shown="True" w606 {
                      tunnel: w607 -> [_ w629]
                      frame False {
                      }
                      frame True {
                        n740 = Get Date/Time In Seconds() -> (seconds since 1Jan1904=w614:timestamp)
                        n741 = global read "rio_Global.vi" "LCM_GGA_T"() -> (w638:T14)
                        n742 = To Double Precision Float(number=w614) -> (double precision float=w613:dbl)
                        n743 = Array To Cluster(array=w629) -> (cluster=w637:T15)
                        n744 = Unbundle By Name(w638) -> ("hash"=w634:i64)
                        n745 = Multiply(x=w613, y=1000000.0) -> (x*y=w611:dbl)
                        n746 = Unbundle(w637) -> ("output[0]"=w639:dbl, "output[2]"=w628:dbl, "output[3]"=w627:dbl, "output[4]"=w626:dbl, "output[6]"=w625:dbl, "output[7]"=w623:dbl, "output[8]"=w621:dbl, "output[9]"=w619:dbl, "output[12]"=w618:dbl, "output[13]"=w617:dbl, "output[14]"=w616:dbl)  [unwired: 4 out]
                        n747 = call "hash.vi"("input"=w634) -> ("output"=w633:i64)  [unwired: 10 in]
                        n748 = To Quad Integer(1:w611) -> (0:w610:i64)
                        n749 = To Long Integer(number=w625) -> (32bit integer=w624:i32)
                        n750 = To Long Integer(number=w623) -> (32bit integer=w622:i32)
                        n751 = To Long Integer(number=w621) -> (32bit integer=w620:i32)
                        n752 = local read "map"() -> (w615:i32)
                        n753 = Bundle(cluster=w638, "hash"=w633, "sys time"=w610, "time"=w639, "x"=w628, "y"=w627, "h"=w626, "numSV"=w624, "postype"=w622, "lag"=w620, "hordev"=w619, "lat"=w618, "lon"=w617, "hgt"=w616, "map_idx"=w615) -> (w635:T14)
                        n754 = Flatten To String(anything=w635, prepend array or string size? (T)=FALSE) -> (data string=w631:string)  [unwired: 2 in, 2 out]
                        n755 = global read "rio_Global.vi" "LCM"() -> (w630:T4)
                        n756 = call "LCM_send.vi"("DATA"=w631, "ID"="GGA_1", "LCM"=w630) -> ()  [unwired: 7 in, 2 out]
                      }
                    }
                  }
                  frame 2 {
                    n757 = flat-sequence {
                      tunnel: w640 -> [w642]
                      frame #0 {
                        n758 = Index Array(array=w642, index=1) -> (element=w644:dbl)
                        n759 = Not Equal To 0?(x=w644) -> (x != 0?=w641:bool)
                        n760 = case shown="True" w641 {
                          tunnel: w642 -> [_ w663]
                          frame False {
                          }
                          frame True {
                            n761 = Get Date/Time In Seconds() -> (seconds since 1Jan1904=w649:timestamp)
                            n762 = To Double Precision Float(number=w649) -> (double precision float=w648:dbl)
                            n763 = global read "rio_Global.vi" "LCM_RMC_T"() -> (w664:T16)
                            n764 = Unbundle By Name(w664) -> ("hash"=w660:i64)
                            n765 = Multiply(x=w648, y=1000000.0) -> (x*y=w646:dbl)
                            n766 = Array To Cluster(array=w663) -> (cluster=w662:T17)
                            n767 = To Quad Integer(1:w646) -> (0:w645:i64)
                            n768 = call "hash.vi"("input"=w660) -> ("output"=w659:i64)  [unwired: 10 in]
                            n769 = Unbundle(w662) -> ("output[0]"=w654:dbl, "output[2]"=w653:dbl, "output[4]"=w652:dbl, "output[5]"=w651:dbl, "output[6]"=w650:dbl)  [unwired: 2 out]
                            n770 = Bundle(cluster=w664, "hash"=w659, "sys time"=w645, "time"=w654, "speed"=w653, "heading"=w652, "lat"=w651, "lon"=w650) -> (w655:T16)
                            n771 = Flatten To String(anything=w655, prepend array or string size? (T)=FALSE) -> (data string=w657:string)  [unwired: 2 in, 2 out]
                            n772 = global read "rio_Global.vi" "LCM"() -> (w656:T4)
                            n773 = call "LCM_send.vi"("DATA"=w657, "ID"="RMC_1", "LCM"=w656) -> ()  [unwired: 7 in, 2 out]
                          }
                        }
                      }
                    }
                    n774 = global write "rio_Global.vi" "gps_vel 1"(w640) -> ()
                  }
                }
              }
            }
          }
        }
      }
    }
  }
